vi "4 en linea.vi"() -> ()   [LabVIEW 2021]
panel:
  in  "OK Button":bool
  out "verde":bool
  in  "col7":bool
  in  "col6":bool
  in  "col5":bool
  in  "col4":bool
  in  "col3":bool
  in  "col2":bool
  in  "col1":bool
  in  "Ring 42":u16(ring)
  in  "Ring 41":u16(ring)
  in  "Ring 40":u16(ring)
  in  "Ring 39":u16(ring)
  in  "Ring 38":u16(ring)
  in  "Ring 37":u16(ring)
  in  "Ring 36":u16(ring)
  in  "Ring 35":u16(ring)
  in  "Ring 34":u16(ring)
  in  "Ring 33":u16(ring)
  in  "Ring 32":u16(ring)
  in  "Ring 31":u16(ring)
  in  "Ring 30":u16(ring)
  in  "Ring 29":u16(ring)
  in  "Ring 28":u16(ring)
  in  "Ring 27":u16(ring)
  in  "Ring 26":u16(ring)
  in  "Ring 25":u16(ring)
  in  "Ring 24":u16(ring)
  in  "Ring 23":u16(ring)
  in  "Ring 22":u16(ring)
  in  "Ring 21":u16(ring)
  in  "Ring 20":u16(ring)
  in  "Ring 19":u16(ring)
  in  "Ring 18":u16(ring)
  in  "Ring 17":u16(ring)
  in  "Ring 16":u16(ring)
  in  "Ring 15":u16(ring)
  in  "Ring 14":u16(ring)
  in  "Ring 13":u16(ring)
  in  "Ring 12":u16(ring)
  in  "Ring 11":u16(ring)
  in  "Ring 10":u16(ring)
  in  "Ring 9":u16(ring)
  in  "Ring 8":u16(ring)
  in  "Ring 7":u16(ring)
  in  "Ring 6":u16(ring)
  in  "Ring 5":u16(ring)
  in  "Ring 4":u16(ring)
  in  "Ring 3":u16(ring)
  in  "Ring 2":u16(ring)
  in  "Ring 1":u16(ring)
  # "4 EN LINEA"
  # "TURNO"
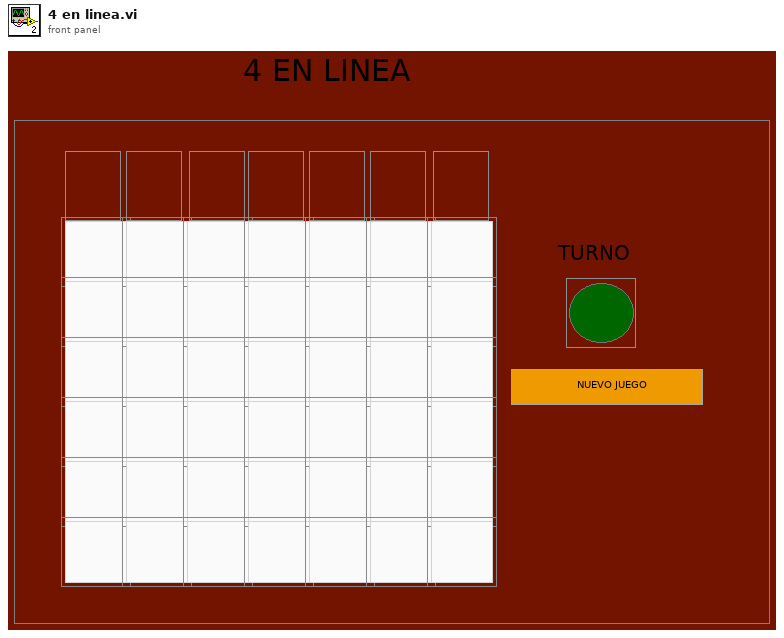
[diagram p1: front panel]
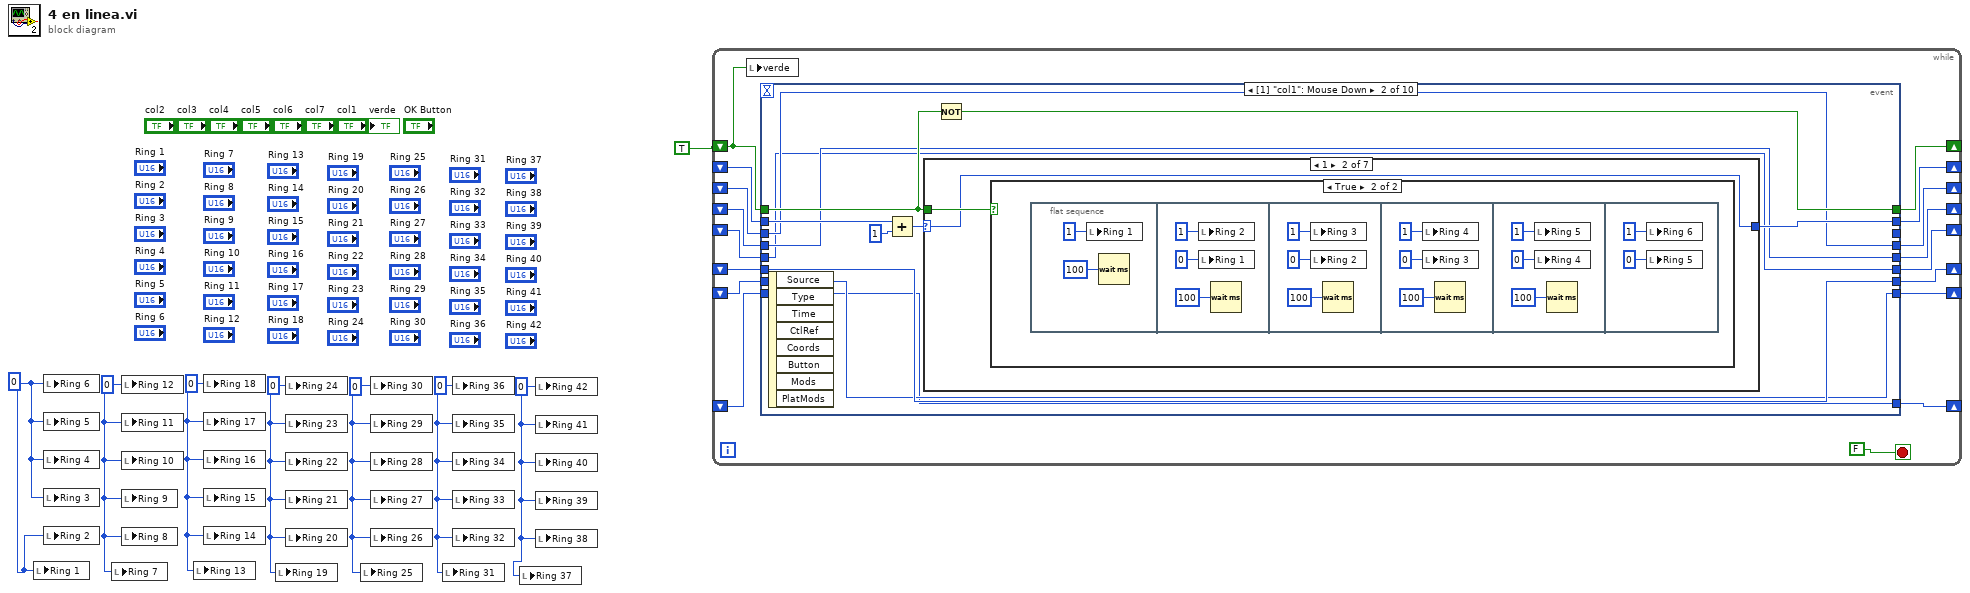
[diagram p0: block diagram]
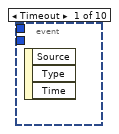
[diagram p2: hidden frame]
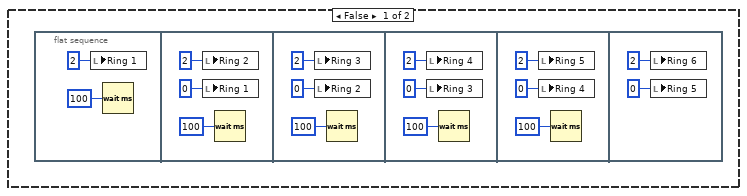
[diagram p4: hidden frame]
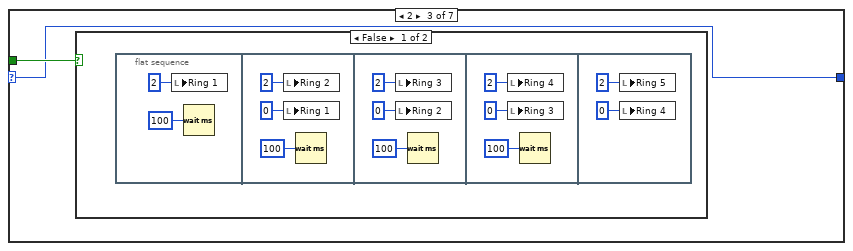
[diagram p5: hidden frame]
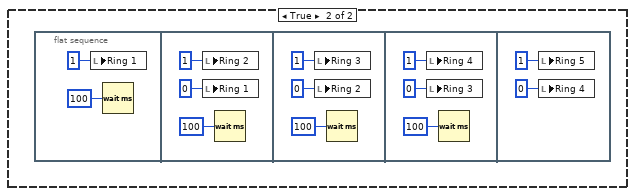
[diagram p6: hidden frame]
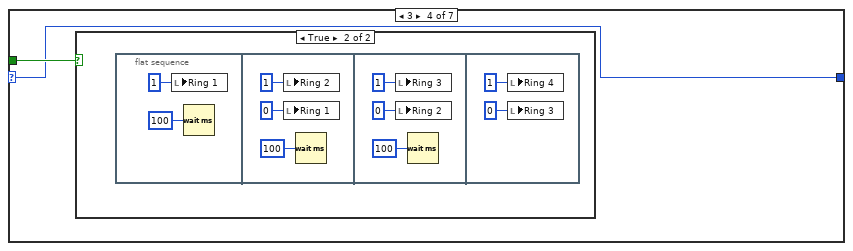
[diagram p7: hidden frame]
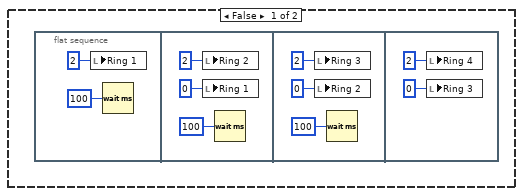
[diagram p8: hidden frame]
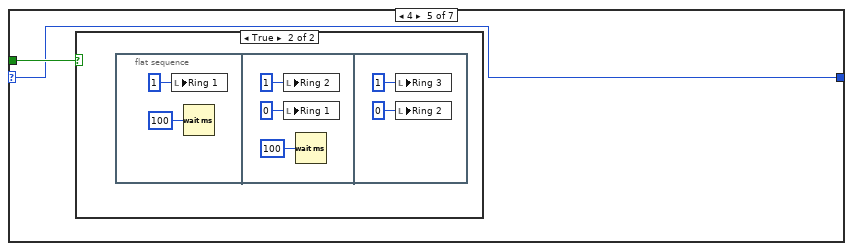
[diagram p9: hidden frame]
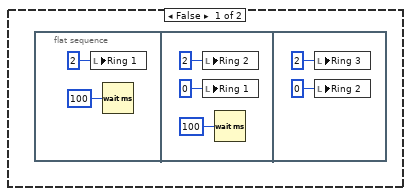
[diagram p10: hidden frame]
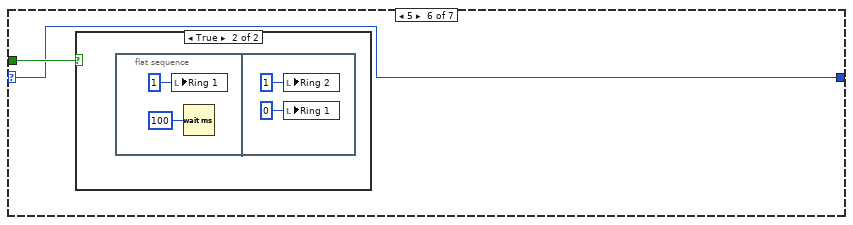
[diagram p11: hidden frame]
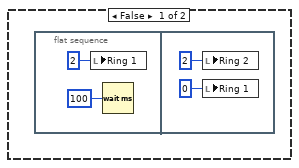
[diagram p12: hidden frame]
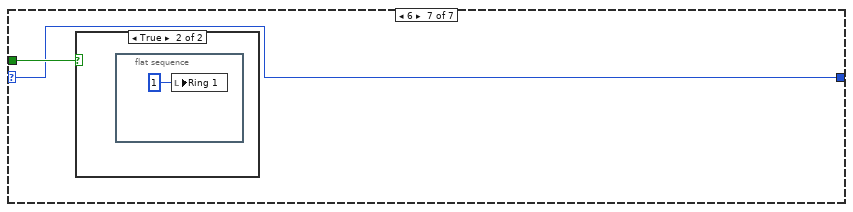
[diagram p13: hidden frame]
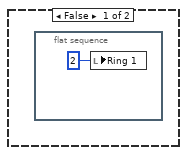
[diagram p14: hidden frame]
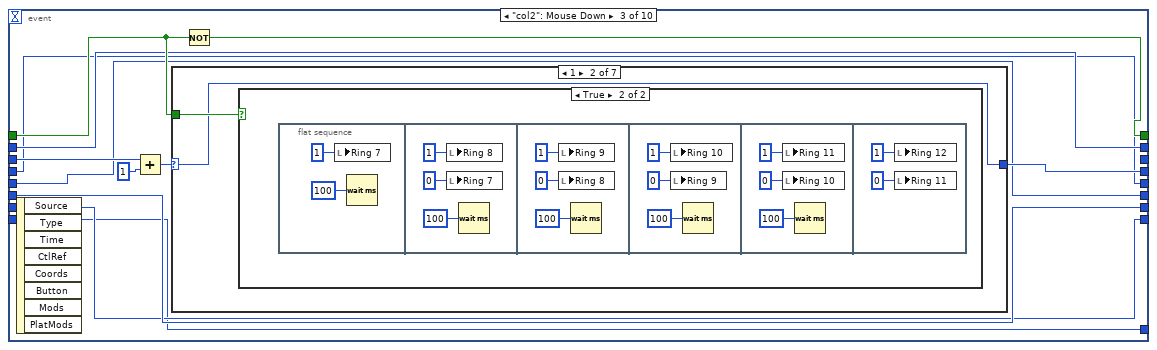
[diagram p15: hidden frame]
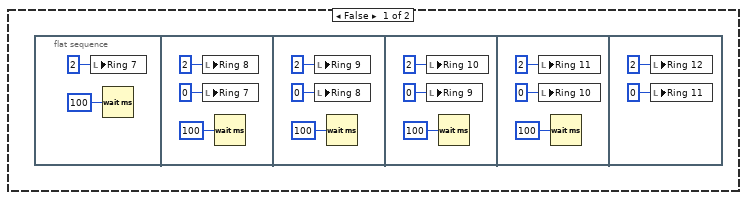
[diagram p17: hidden frame]
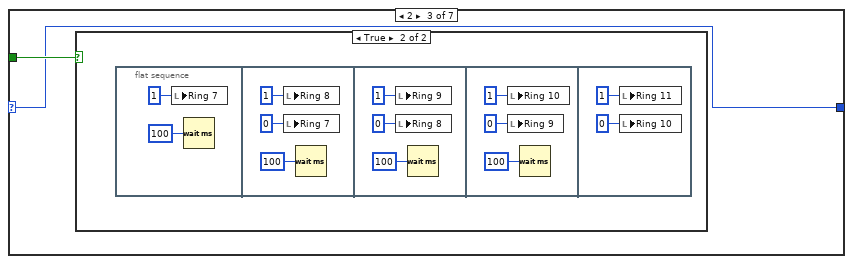
[diagram p18: hidden frame]
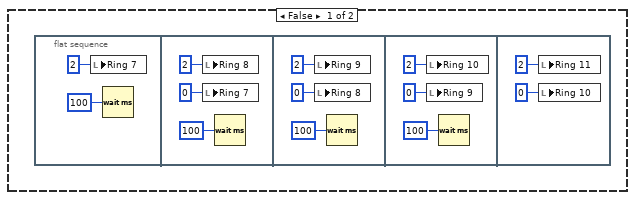
[diagram p19: hidden frame]
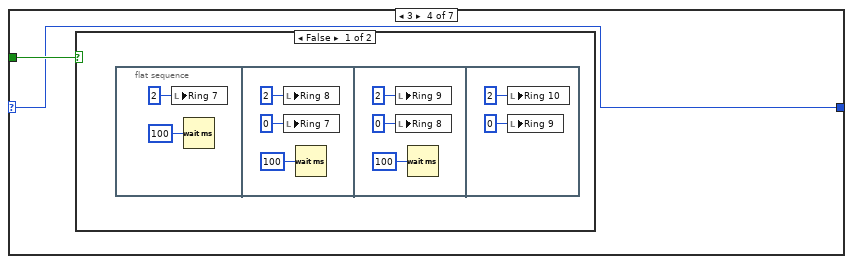
[diagram p20: hidden frame]
diagram:
  w2 = u16 0 ("Ring 42")
  w3 = u16 0 ("Ring 36")
  w4 = u16 0 ("Ring 30")
  w5 = u16 0 ("Ring 24")
  w6 = u16 0 ("Ring 18")
  w7 = u16 0 ("Ring 12")
  w8 = 0
  n1 = local write "Ring 1"(w8) -> ()
  n2 = local write "Ring 6"(w8) -> ()
  n3 = local write "Ring 5"(w8) -> ()
  n4 = local write "Ring 4"(w8) -> ()
  n5 = local write "Ring 3"(w8) -> ()
  n6 = local write "Ring 2"(w8) -> ()
  n7 = local write "Ring 7"(w7) -> ()
  n8 = local write "Ring 12"(w7) -> ()
  n9 = local write "Ring 11"(w7) -> ()
  n10 = local write "Ring 10"(w7) -> ()
  n11 = local write "Ring 9"(w7) -> ()
  n12 = local write "Ring 8"(w7) -> ()
  n13 = local write "Ring 13"(w6) -> ()
  n14 = local write "Ring 18"(w6) -> ()
  n15 = local write "Ring 17"(w6) -> ()
  n16 = local write "Ring 16"(w6) -> ()
  n17 = local write "Ring 15"(w6) -> ()
  n18 = local write "Ring 14"(w6) -> ()
  n19 = local write "Ring 19"(w5) -> ()
  n20 = local write "Ring 24"(w5) -> ()
  n21 = local write "Ring 23"(w5) -> ()
  n22 = local write "Ring 22"(w5) -> ()
  n23 = local write "Ring 21"(w5) -> ()
  n24 = local write "Ring 20"(w5) -> ()
  n25 = local write "Ring 25"(w4) -> ()
  n26 = local write "Ring 30"(w4) -> ()
  n27 = local write "Ring 29"(w4) -> ()
  n28 = local write "Ring 28"(w4) -> ()
  n29 = local write "Ring 27"(w4) -> ()
  n30 = local write "Ring 26"(w4) -> ()
  n31 = local write "Ring 31"(w3) -> ()
  n32 = local write "Ring 36"(w3) -> ()
  n33 = local write "Ring 35"(w3) -> ()
  n34 = local write "Ring 34"(w3) -> ()
  n35 = local write "Ring 33"(w3) -> ()
  n36 = local write "Ring 32"(w3) -> ()
  n37 = local write "Ring 37"(w2) -> ()
  n38 = local write "Ring 42"(w2) -> ()
  n39 = local write "Ring 41"(w2) -> ()
  n40 = local write "Ring 40"(w2) -> ()
  n41 = local write "Ring 39"(w2) -> ()
  n42 = local write "Ring 38"(w2) -> ()
  n43 = while {
    shift-right: [w24] -> _
    shift-left: TRUE -> [w9]
    shift-right: [w23] -> _
    shift-left: _ -> [w21]
    shift-right: [w22] -> _
    shift-left: _ -> [w20]
    shift-right: [w19] -> _
    shift-left: _ -> [w17]
    shift-right: [w18] -> _
    shift-left: _ -> [w16]
    shift-right: [w14] -> _
    shift-left: _ -> [w15]
    shift-right: [w12] -> _
    shift-left: _ -> [w13]
    shift-right: [w10] -> _
    shift-left: _ -> [w11]
    stop <- FALSE stop-if-true
    n44 = local write "verde"(w9) -> ()
    n45 = event shown="[1] \"col1\": Mouse Down" {
      selector: _ -> [_ _ _ _ _ _ _ _ _ _]
      dyn-events: _ -> [_ _ _ _ _ _ _ _ _ _]
      timeout: _ -> [_ _ _ _ _ _ _ _ _ _]
      tunnel: w9 -> [_ w36 w163 w285 w411 w540 w668 w788 w915 _]
      tunnel: [_ w37 w164 w286 w410 w541 w667 w789 w915 _] -> w24
      tunnel: [_ w35 w158 w289 w414 w536 w666 w795 _ _] -> w23
      tunnel: [_ w31 w162 w290 w413 w537 w665 w794 w921 _] -> w22
      tunnel: w21 -> [_ w34 w158 w289 w414 w536 w666 w795 w922 _]
      tunnel: w20 -> [_ w31 w161 w290 w413 w537 w665 w794 w921 _]
      tunnel: [_ w30 w157 w291 w412 w538 w664 w793 w920 _] -> w19
      tunnel: [_ w29 w156 w283 w416 w539 w663 w792 w919 _] -> w18
      tunnel: w17 -> [_ w30 w157 w284 w412 w538 w664 w793 w920 _]
      tunnel: w16 -> [_ w29 w156 w283 w415 w539 w663 w792 w919 _]
      tunnel: w15 -> [_ w28 w155 w282 w409 w544 w662 w791 w918 _]
      tunnel: [_ w28 w155 w282 w409 w542 w662 w791 w918 _] -> w14
      tunnel: w13 -> [_ w27 w154 w281 w408 w535 w671 w790 w917 _]
      tunnel: [_ w27 w154 w281 w408 w535 w669 w790 w917 _] -> w12
      tunnel: w11 -> [_ w26 w153 w280 w407 w534 w661 w798 w916 _]
      tunnel: [_ w26 w153 w280 w407 w534 w661 w796 w916 _] -> w10
      tunnel: [_ _ _ _ _ _ _ _ w922 _] -> _
      event Timeout {
        n46 = event-data() -> ()  [unwired: 1 in, 3 out]
      }
      event "col1": Mouse Down {
        n47 = event-data() -> ()  [unwired: 1 in, 8 out]
        n48 = Add(x=w34, y=1) -> (x+y=w33:i32)
        n49 = case shown="1" w33 {
          selector: w33 -> [w38 w39 w73 w101 w123 w139 w149]
          tunnel: w36 -> [_ w40 w74 w102 w124 w140 w150]
          tunnel: [w38 w39 w73 w101 w123 w139 w149] -> w35
          frame 0, Default {
          }
          frame 1 {
            n50 = case shown="True" w40 {
              frame False {
                n51 = flat-sequence {
                  frame #0 {
                    n52 = local write "Ring 1"(u16 2 ("Ring 1")) -> ()
                    n53 = Wait (ms)(milliseconds to wait=u32 100) -> ()  [unwired: 1 out]
                  }
                  frame #1 {
                    n54 = local write "Ring 2"(u16 2 ("Ring 2")) -> ()
                    n55 = local write "Ring 1"(u16 0 ("Ring 1")) -> ()
                    n56 = Wait (ms)(milliseconds to wait=u32 100) -> ()  [unwired: 1 out]
                  }
                  frame #2 {
                    n57 = local write "Ring 3"(u16 2 ("Ring 3")) -> ()
                    n58 = local write "Ring 2"(u16 0 ("Ring 2")) -> ()
                    n59 = Wait (ms)(milliseconds to wait=u32 100) -> ()  [unwired: 1 out]
                  }
                  frame #3 {
                    n60 = local write "Ring 4"(u16 2 ("Ring 4")) -> ()
                    n61 = local write "Ring 3"(u16 0 ("Ring 3")) -> ()
                    n62 = Wait (ms)(milliseconds to wait=u32 100) -> ()  [unwired: 1 out]
                  }
                  frame #4 {
                    n63 = local write "Ring 5"(u16 2 ("Ring 5")) -> ()
                    n64 = local write "Ring 4"(u16 0 ("Ring 4")) -> ()
                    n65 = Wait (ms)(milliseconds to wait=u32 100) -> ()  [unwired: 1 out]
                  }
                  frame #5 {
                    n66 = local write "Ring 6"(u16 2 ("Ring 6")) -> ()
                    n67 = local write "Ring 5"(u16 0 ("Ring 5")) -> ()
                  }
                }
              }
              frame True {
                n68 = flat-sequence {
                  frame #0 {
                    n69 = local write "Ring 1"(u16 1 ("Ring 1")) -> ()
                    n70 = Wait (ms)(milliseconds to wait=u32 100) -> ()  [unwired: 1 out]
                  }
                  frame #1 {
                    n71 = local write "Ring 2"(u16 1 ("Ring 2")) -> ()
                    n72 = local write "Ring 1"(u16 0 ("Ring 1")) -> ()
                    n73 = Wait (ms)(milliseconds to wait=u32 100) -> ()  [unwired: 1 out]
                  }
                  frame #2 {
                    n74 = local write "Ring 3"(u16 1 ("Ring 3")) -> ()
                    n75 = local write "Ring 2"(u16 0 ("Ring 2")) -> ()
                    n76 = Wait (ms)(milliseconds to wait=u32 100) -> ()  [unwired: 1 out]
                  }
                  frame #3 {
                    n77 = local write "Ring 4"(u16 1 ("Ring 4")) -> ()
                    n78 = local write "Ring 3"(u16 0 ("Ring 3")) -> ()
                    n79 = Wait (ms)(milliseconds to wait=u32 100) -> ()  [unwired: 1 out]
                  }
                  frame #4 {
                    n80 = local write "Ring 5"(u16 1 ("Ring 5")) -> ()
                    n81 = local write "Ring 4"(u16 0 ("Ring 4")) -> ()
                    n82 = Wait (ms)(milliseconds to wait=u32 100) -> ()  [unwired: 1 out]
                  }
                  frame #5 {
                    n83 = local write "Ring 6"(u16 1 ("Ring 6")) -> ()
                    n84 = local write "Ring 5"(u16 0 ("Ring 5")) -> ()
                  }
                }
              }
            }
          }
          frame 2 {
            n85 = case shown="False" w74 {
              frame False {
                n86 = flat-sequence {
                  frame #0 {
                    n87 = local write "Ring 1"(u16 2 ("Ring 1")) -> ()
                    n88 = Wait (ms)(milliseconds to wait=u32 100) -> ()  [unwired: 1 out]
                  }
                  frame #1 {
                    n89 = local write "Ring 2"(u16 2 ("Ring 2")) -> ()
                    n90 = local write "Ring 1"(u16 0 ("Ring 1")) -> ()
                    n91 = Wait (ms)(milliseconds to wait=u32 100) -> ()  [unwired: 1 out]
                  }
                  frame #2 {
                    n92 = local write "Ring 3"(u16 2 ("Ring 3")) -> ()
                    n93 = local write "Ring 2"(u16 0 ("Ring 2")) -> ()
                    n94 = Wait (ms)(milliseconds to wait=u32 100) -> ()  [unwired: 1 out]
                  }
                  frame #3 {
                    n95 = local write "Ring 4"(u16 2 ("Ring 4")) -> ()
                    n96 = local write "Ring 3"(u16 0 ("Ring 3")) -> ()
                    n97 = Wait (ms)(milliseconds to wait=u32 100) -> ()  [unwired: 1 out]
                  }
                  frame #4 {
                    n98 = local write "Ring 5"(u16 2 ("Ring 5")) -> ()
                    n99 = local write "Ring 4"(u16 0 ("Ring 4")) -> ()
                  }
                }
              }
              frame True {
                n100 = flat-sequence {
                  frame #0 {
                    n101 = local write "Ring 1"(u16 1 ("Ring 1")) -> ()
                    n102 = Wait (ms)(milliseconds to wait=u32 100) -> ()  [unwired: 1 out]
                  }
                  frame #1 {
                    n103 = local write "Ring 2"(u16 1 ("Ring 2")) -> ()
                    n104 = local write "Ring 1"(u16 0 ("Ring 1")) -> ()
                    n105 = Wait (ms)(milliseconds to wait=u32 100) -> ()  [unwired: 1 out]
                  }
                  frame #2 {
                    n106 = local write "Ring 3"(u16 1 ("Ring 3")) -> ()
                    n107 = local write "Ring 2"(u16 0 ("Ring 2")) -> ()
                    n108 = Wait (ms)(milliseconds to wait=u32 100) -> ()  [unwired: 1 out]
                  }
                  frame #3 {
                    n109 = local write "Ring 4"(u16 1 ("Ring 4")) -> ()
                    n110 = local write "Ring 3"(u16 0 ("Ring 3")) -> ()
                    n111 = Wait (ms)(milliseconds to wait=u32 100) -> ()  [unwired: 1 out]
                  }
                  frame #4 {
                    n112 = local write "Ring 5"(u16 1 ("Ring 5")) -> ()
                    n113 = local write "Ring 4"(u16 0 ("Ring 4")) -> ()
                  }
                }
              }
            }
          }
          frame 3 {
            n114 = case shown="True" w102 {
              frame False {
                n115 = flat-sequence {
                  frame #0 {
                    n116 = local write "Ring 1"(u16 2 ("Ring 1")) -> ()
                    n117 = Wait (ms)(milliseconds to wait=u32 100) -> ()  [unwired: 1 out]
                  }
                  frame #1 {
                    n118 = local write "Ring 2"(u16 2 ("Ring 2")) -> ()
                    n119 = local write "Ring 1"(u16 0 ("Ring 1")) -> ()
                    n120 = Wait (ms)(milliseconds to wait=u32 100) -> ()  [unwired: 1 out]
                  }
                  frame #2 {
                    n121 = local write "Ring 3"(u16 2 ("Ring 3")) -> ()
                    n122 = local write "Ring 2"(u16 0 ("Ring 2")) -> ()
                    n123 = Wait (ms)(milliseconds to wait=u32 100) -> ()  [unwired: 1 out]
                  }
                  frame #3 {
                    n124 = local write "Ring 4"(u16 2 ("Ring 4")) -> ()
                    n125 = local write "Ring 3"(u16 0 ("Ring 3")) -> ()
                  }
                }
              }
              frame True {
                n126 = flat-sequence {
                  frame #0 {
                    n127 = local write "Ring 1"(u16 1 ("Ring 1")) -> ()
                    n128 = Wait (ms)(milliseconds to wait=u32 100) -> ()  [unwired: 1 out]
                  }
                  frame #1 {
                    n129 = local write "Ring 2"(u16 1 ("Ring 2")) -> ()
                    n130 = local write "Ring 1"(u16 0 ("Ring 1")) -> ()
                    n131 = Wait (ms)(milliseconds to wait=u32 100) -> ()  [unwired: 1 out]
                  }
                  frame #2 {
                    n132 = local write "Ring 3"(u16 1 ("Ring 3")) -> ()
                    n133 = local write "Ring 2"(u16 0 ("Ring 2")) -> ()
                    n134 = Wait (ms)(milliseconds to wait=u32 100) -> ()  [unwired: 1 out]
                  }
                  frame #3 {
                    n135 = local write "Ring 4"(u16 1 ("Ring 4")) -> ()
                    n136 = local write "Ring 3"(u16 0 ("Ring 3")) -> ()
                  }
                }
              }
            }
          }
          frame 4 {
            n137 = case shown="True" w124 {
              frame False {
                n138 = flat-sequence {
                  frame #0 {
                    n139 = local write "Ring 1"(u16 2 ("Ring 1")) -> ()
                    n140 = Wait (ms)(milliseconds to wait=u32 100) -> ()  [unwired: 1 out]
                  }
                  frame #1 {
                    n141 = local write "Ring 2"(u16 2 ("Ring 2")) -> ()
                    n142 = local write "Ring 1"(u16 0 ("Ring 1")) -> ()
                    n143 = Wait (ms)(milliseconds to wait=u32 100) -> ()  [unwired: 1 out]
                  }
                  frame #2 {
                    n144 = local write "Ring 3"(u16 2 ("Ring 3")) -> ()
                    n145 = local write "Ring 2"(u16 0 ("Ring 2")) -> ()
                  }
                }
              }
              frame True {
                n146 = flat-sequence {
                  frame #0 {
                    n147 = local write "Ring 1"(u16 1 ("Ring 1")) -> ()
                    n148 = Wait (ms)(milliseconds to wait=u32 100) -> ()  [unwired: 1 out]
                  }
                  frame #1 {
                    n149 = local write "Ring 2"(u16 1 ("Ring 2")) -> ()
                    n150 = local write "Ring 1"(u16 0 ("Ring 1")) -> ()
                    n151 = Wait (ms)(milliseconds to wait=u32 100) -> ()  [unwired: 1 out]
                  }
                  frame #2 {
                    n152 = local write "Ring 3"(u16 1 ("Ring 3")) -> ()
                    n153 = local write "Ring 2"(u16 0 ("Ring 2")) -> ()
                  }
                }
              }
            }
          }
          frame 5 {
            n154 = case shown="True" w140 {
              frame False {
                n155 = flat-sequence {
                  frame #0 {
                    n156 = local write "Ring 1"(u16 2 ("Ring 1")) -> ()
                    n157 = Wait (ms)(milliseconds to wait=u32 100) -> ()  [unwired: 1 out]
                  }
                  frame #1 {
                    n158 = local write "Ring 2"(u16 2 ("Ring 2")) -> ()
                    n159 = local write "Ring 1"(u16 0 ("Ring 1")) -> ()
                  }
                }
              }
              frame True {
                n160 = flat-sequence {
                  frame #0 {
                    n161 = local write "Ring 1"(u16 1 ("Ring 1")) -> ()
                    n162 = Wait (ms)(milliseconds to wait=u32 100) -> ()  [unwired: 1 out]
                  }
                  frame #1 {
                    n163 = local write "Ring 2"(u16 1 ("Ring 2")) -> ()
                    n164 = local write "Ring 1"(u16 0 ("Ring 1")) -> ()
                  }
                }
              }
            }
          }
          frame 6 {
            n165 = case shown="True" w150 {
              frame False {
                n166 = flat-sequence {
                  frame #0 {
                    n167 = local write "Ring 1"(u16 2 ("Ring 1")) -> ()
                  }
                }
              }
              frame True {
                n168 = flat-sequence {
                  frame #0 {
                    n169 = local write "Ring 1"(u16 1 ("Ring 1")) -> ()
                  }
                }
              }
            }
          }
        }
        n170 = Not(x=w36) -> (.not. x?=w37:bool)
      }
      event "col2": Mouse Down {
        n171 = event-data() -> ()  [unwired: 1 in, 8 out]
        n172 = Add(x=w161, y=1) -> (x+y=w160:i32)
        n173 = case shown="1" w160 {
          selector: w160 -> [w165 w166 w200 w228 w250 w266 w276]
          tunnel: w163 -> [_ w167 w201 w229 w251 w267 w277]
          tunnel: [w165 w166 w200 w228 w250 w266 w276] -> w162
          frame 0, Default {
          }
          frame 1 {
            n174 = case shown="True" w167 {
              frame False {
                n175 = flat-sequence {
                  frame #0 {
                    n176 = local write "Ring 7"(u16 2 ("Ring 1")) -> ()
                    n177 = Wait (ms)(milliseconds to wait=u32 100) -> ()  [unwired: 1 out]
                  }
                  frame #1 {
                    n178 = local write "Ring 8"(u16 2 ("Ring 2")) -> ()
                    n179 = local write "Ring 7"(u16 0 ("Ring 1")) -> ()
                    n180 = Wait (ms)(milliseconds to wait=u32 100) -> ()  [unwired: 1 out]
                  }
                  frame #2 {
                    n181 = local write "Ring 9"(u16 2 ("Ring 3")) -> ()
                    n182 = local write "Ring 8"(u16 0 ("Ring 2")) -> ()
                    n183 = Wait (ms)(milliseconds to wait=u32 100) -> ()  [unwired: 1 out]
                  }
                  frame #3 {
                    n184 = local write "Ring 10"(u16 2 ("Ring 4")) -> ()
                    n185 = local write "Ring 9"(u16 0 ("Ring 3")) -> ()
                    n186 = Wait (ms)(milliseconds to wait=u32 100) -> ()  [unwired: 1 out]
                  }
                  frame #4 {
                    n187 = local write "Ring 11"(u16 2 ("Ring 5")) -> ()
                    n188 = local write "Ring 10"(u16 0 ("Ring 4")) -> ()
                    n189 = Wait (ms)(milliseconds to wait=u32 100) -> ()  [unwired: 1 out]
                  }
                  frame #5 {
                    n190 = local write "Ring 12"(u16 2 ("Ring 6")) -> ()
                    n191 = local write "Ring 11"(u16 0 ("Ring 5")) -> ()
                  }
                }
              }
              frame True {
                n192 = flat-sequence {
                  frame #0 {
                    n193 = local write "Ring 7"(u16 1 ("Ring 1")) -> ()
                    n194 = Wait (ms)(milliseconds to wait=u32 100) -> ()  [unwired: 1 out]
                  }
                  frame #1 {
                    n195 = local write "Ring 8"(u16 1 ("Ring 2")) -> ()
                    n196 = local write "Ring 7"(u16 0 ("Ring 1")) -> ()
                    n197 = Wait (ms)(milliseconds to wait=u32 100) -> ()  [unwired: 1 out]
                  }
                  frame #2 {
                    n198 = local write "Ring 9"(u16 1 ("Ring 3")) -> ()
                    n199 = local write "Ring 8"(u16 0 ("Ring 2")) -> ()
                    n200 = Wait (ms)(milliseconds to wait=u32 100) -> ()  [unwired: 1 out]
                  }
                  frame #3 {
                    n201 = local write "Ring 10"(u16 1 ("Ring 4")) -> ()
                    n202 = local write "Ring 9"(u16 0 ("Ring 3")) -> ()
                    n203 = Wait (ms)(milliseconds to wait=u32 100) -> ()  [unwired: 1 out]
                  }
                  frame #4 {
                    n204 = local write "Ring 11"(u16 1 ("Ring 5")) -> ()
                    n205 = local write "Ring 10"(u16 0 ("Ring 4")) -> ()
                    n206 = Wait (ms)(milliseconds to wait=u32 100) -> ()  [unwired: 1 out]
                  }
                  frame #5 {
                    n207 = local write "Ring 12"(u16 1 ("Ring 6")) -> ()
                    n208 = local write "Ring 11"(u16 0 ("Ring 5")) -> ()
                  }
                }
              }
            }
          }
          frame 2 {
            n209 = case shown="True" w201 {
              frame False {
                n210 = flat-sequence {
                  frame #0 {
                    n211 = local write "Ring 7"(u16 2 ("Ring 1")) -> ()
                    n212 = Wait (ms)(milliseconds to wait=u32 100) -> ()  [unwired: 1 out]
                  }
                  frame #1 {
                    n213 = local write "Ring 8"(u16 2 ("Ring 2")) -> ()
                    n214 = local write "Ring 7"(u16 0 ("Ring 1")) -> ()
                    n215 = Wait (ms)(milliseconds to wait=u32 100) -> ()  [unwired: 1 out]
                  }
                  frame #2 {
                    n216 = local write "Ring 9"(u16 2 ("Ring 3")) -> ()
                    n217 = local write "Ring 8"(u16 0 ("Ring 2")) -> ()
                    n218 = Wait (ms)(milliseconds to wait=u32 100) -> ()  [unwired: 1 out]
                  }
                  frame #3 {
                    n219 = local write "Ring 10"(u16 2 ("Ring 4")) -> ()
                    n220 = local write "Ring 9"(u16 0 ("Ring 3")) -> ()
                    n221 = Wait (ms)(milliseconds to wait=u32 100) -> ()  [unwired: 1 out]
                  }
                  frame #4 {
                    n222 = local write "Ring 11"(u16 2 ("Ring 5")) -> ()
                    n223 = local write "Ring 10"(u16 0 ("Ring 4")) -> ()
                  }
                }
              }
              frame True {
                n224 = flat-sequence {
                  frame #0 {
                    n225 = local write "Ring 7"(u16 1 ("Ring 1")) -> ()
                    n226 = Wait (ms)(milliseconds to wait=u32 100) -> ()  [unwired: 1 out]
                  }
                  frame #1 {
                    n227 = local write "Ring 8"(u16 1 ("Ring 2")) -> ()
                    n228 = local write "Ring 7"(u16 0 ("Ring 1")) -> ()
                    n229 = Wait (ms)(milliseconds to wait=u32 100) -> ()  [unwired: 1 out]
                  }
                  frame #2 {
                    n230 = local write "Ring 9"(u16 1 ("Ring 3")) -> ()
                    n231 = local write "Ring 8"(u16 0 ("Ring 2")) -> ()
                    n232 = Wait (ms)(milliseconds to wait=u32 100) -> ()  [unwired: 1 out]
                  }
                  frame #3 {
                    n233 = local write "Ring 10"(u16 1 ("Ring 4")) -> ()
                    n234 = local write "Ring 9"(u16 0 ("Ring 3")) -> ()
                    n235 = Wait (ms)(milliseconds to wait=u32 100) -> ()  [unwired: 1 out]
                  }
                  frame #4 {
                    n236 = local write "Ring 11"(u16 1 ("Ring 5")) -> ()
                    n237 = local write "Ring 10"(u16 0 ("Ring 4")) -> ()
                  }
                }
              }
            }
          }
          frame 3 {
            n238 = case shown="False" w229 {
              frame False {
                n239 = flat-sequence {
                  frame #0 {
                    n240 = local write "Ring 7"(u16 2 ("Ring 1")) -> ()
                    n241 = Wait (ms)(milliseconds to wait=u32 100) -> ()  [unwired: 1 out]
                  }
                  frame #1 {
                    n242 = local write "Ring 8"(u16 2 ("Ring 2")) -> ()
                    n243 = local write "Ring 7"(u16 0 ("Ring 1")) -> ()
                    n244 = Wait (ms)(milliseconds to wait=u32 100) -> ()  [unwired: 1 out]
                  }
                  frame #2 {
                    n245 = local write "Ring 9"(u16 2 ("Ring 3")) -> ()
                    n246 = local write "Ring 8"(u16 0 ("Ring 2")) -> ()
                    n247 = Wait (ms)(milliseconds to wait=u32 100) -> ()  [unwired: 1 out]
                  }
                  frame #3 {
                    n248 = local write "Ring 10"(u16 2 ("Ring 4")) -> ()
                    n249 = local write "Ring 9"(u16 0 ("Ring 3")) -> ()
                  }
                }
              }
              frame True {
                n250 = flat-sequence {
                  frame #0 {
                    n251 = local write "Ring 7"(u16 1 ("Ring 1")) -> ()
                    n252 = Wait (ms)(milliseconds to wait=u32 100) -> ()  [unwired: 1 out]
                  }
                  frame #1 {
                    n253 = local write "Ring 8"(u16 1 ("Ring 2")) -> ()
                    n254 = local write "Ring 7"(u16 0 ("Ring 1")) -> ()
                    n255 = Wait (ms)(milliseconds to wait=u32 100) -> ()  [unwired: 1 out]
                  }
                  frame #2 {
                    n256 = local write "Ring 9"(u16 1 ("Ring 3")) -> ()
                    n257 = local write "Ring 8"(u16 0 ("Ring 2")) -> ()
                    n258 = Wait (ms)(milliseconds to wait=u32 100) -> ()  [unwired: 1 out]
                  }
                  frame #3 {
                    n259 = local write "Ring 10"(u16 1 ("Ring 4")) -> ()
                    n260 = local write "Ring 9"(u16 0 ("Ring 3")) -> ()
                  }
                }
              }
            }
          }
          frame 4 {
            n261 = case shown="True" w251 {
              frame False {
                n262 = flat-sequence {
                  frame #0 {
                    n263 = local write "Ring 7"(u16 2 ("Ring 1")) -> ()
                    n264 = Wait (ms)(milliseconds to wait=u32 100) -> ()  [unwired: 1 out]
                  }
                  frame #1 {
                    n265 = local write "Ring 8"(u16 2 ("Ring 2")) -> ()
                    n266 = local write "Ring 7"(u16 0 ("Ring 1")) -> ()
                    n267 = Wait (ms)(milliseconds to wait=u32 100) -> ()  [unwired: 1 out]
                  }
                  frame #2 {
                    n268 = local write "Ring 9"(u16 2 ("Ring 3")) -> ()
                    n269 = local write "Ring 8"(u16 0 ("Ring 2")) -> ()
                  }
                }
              }
              frame True {
                n270 = flat-sequence {
                  frame #0 {
                    n271 = local write "Ring 7"(u16 1 ("Ring 1")) -> ()
                    n272 = Wait (ms)(milliseconds to wait=u32 100) -> ()  [unwired: 1 out]
                  }
                  frame #1 {
                    n273 = local write "Ring 8"(u16 1 ("Ring 2")) -> ()
                    n274 = local write "Ring 7"(u16 0 ("Ring 1")) -> ()
                    n275 = Wait (ms)(milliseconds to wait=u32 100) -> ()  [unwired: 1 out]
                  }
                  frame #2 {
                    n276 = local write "Ring 9"(u16 1 ("Ring 3")) -> ()
                    n277 = local write "Ring 8"(u16 0 ("Ring 2")) -> ()
                  }
                }
              }
            }
          }
          frame 5 {
            n278 = case shown="True" w267 {
              frame False {
                n279 = flat-sequence {
                  frame #0 {
                    n280 = local write "Ring 7"(u16 2 ("Ring 1")) -> ()
                    n281 = Wait (ms)(milliseconds to wait=u32 100) -> ()  [unwired: 1 out]
                  }
                  frame #1 {
                    n282 = local write "Ring 8"(u16 2 ("Ring 2")) -> ()
                    n283 = local write "Ring 7"(u16 0 ("Ring 1")) -> ()
                  }
                }
              }
              frame True {
                n284 = flat-sequence {
                  frame #0 {
                    n285 = local write "Ring 7"(u16 1 ("Ring 1")) -> ()
                    n286 = Wait (ms)(milliseconds to wait=u32 100) -> ()  [unwired: 1 out]
                  }
                  frame #1 {
                    n287 = local write "Ring 8"(u16 1 ("Ring 2")) -> ()
                    n288 = local write "Ring 7"(u16 0 ("Ring 1")) -> ()
                  }
                }
              }
            }
          }
          frame 6 {
            n289 = case shown="False" w277 {
              frame False {
                n290 = flat-sequence {
                  frame #0 {
                    n291 = local write "Ring 7"(u16 2 ("Ring 1")) -> ()
                  }
                }
              }
              frame True {
                n292 = flat-sequence {
                  frame #0 {
                    n293 = local write "Ring 7"(u16 1 ("Ring 1")) -> ()
                  }
                }
              }
            }
          }
        }
        n294 = Not(x=w163) -> (.not. x?=w164:bool)
      }
      event "col3": Mouse Down {
        n295 = event-data() -> ()  [unwired: 1 in, 8 out]
        n296 = Add(x=w284, y=1) -> (x+y=w288:i32)
        n297 = case shown="1" w288 {
          selector: w288 -> [w292 w293 w327 w355 w377 w393 w403]
          tunnel: w285 -> [_ w294 w328 w356 w378 w394 w404]
          tunnel: [w292 w293 w327 w355 w377 w393 w403] -> w291
          frame 0, Default {
          }
          frame 1 {
            n298 = case shown="False" w294 {
              frame False {
                n299 = flat-sequence {
                  frame #0 {
                    n300 = local write "Ring 13"(u16 2 ("Ring 1")) -> ()
                    n301 = Wait (ms)(milliseconds to wait=u32 100) -> ()  [unwired: 1 out]
                  }
                  frame #1 {
                    n302 = local write "Ring 14"(u16 2 ("Ring 2")) -> ()
                    n303 = local write "Ring 13"(u16 0 ("Ring 1")) -> ()
                    n304 = Wait (ms)(milliseconds to wait=u32 100) -> ()  [unwired: 1 out]
                  }
                  frame #2 {
                    n305 = local write "Ring 15"(u16 2 ("Ring 3")) -> ()
                    n306 = local write "Ring 14"(u16 0 ("Ring 2")) -> ()
                    n307 = Wait (ms)(milliseconds to wait=u32 100) -> ()  [unwired: 1 out]
                  }
                  frame #3 {
                    n308 = local write "Ring 16"(u16 2 ("Ring 4")) -> ()
                    n309 = local write "Ring 15"(u16 0 ("Ring 3")) -> ()
                    n310 = Wait (ms)(milliseconds to wait=u32 100) -> ()  [unwired: 1 out]
                  }
                  frame #4 {
                    n311 = local write "Ring 17"(u16 2 ("Ring 5")) -> ()
                    n312 = local write "Ring 16"(u16 0 ("Ring 4")) -> ()
                    n313 = Wait (ms)(milliseconds to wait=u32 100) -> ()  [unwired: 1 out]
                  }
                  frame #5 {
                    n314 = local write "Ring 18"(u16 2 ("Ring 6")) -> ()
                    n315 = local write "Ring 17"(u16 0 ("Ring 5")) -> ()
                  }
                }
              }
              frame True {
                n316 = flat-sequence {
                  frame #0 {
                    n317 = local write "Ring 13"(u16 1 ("Ring 1")) -> ()
                    n318 = Wait (ms)(milliseconds to wait=u32 100) -> ()  [unwired: 1 out]
                  }
                  frame #1 {
                    n319 = local write "Ring 14"(u16 1 ("Ring 2")) -> ()
                    n320 = local write "Ring 13"(u16 0 ("Ring 1")) -> ()
                    n321 = Wait (ms)(milliseconds to wait=u32 100) -> ()  [unwired: 1 out]
                  }
                  frame #2 {
                    n322 = local write "Ring 15"(u16 1 ("Ring 3")) -> ()
                    n323 = local write "Ring 14"(u16 0 ("Ring 2")) -> ()
                    n324 = Wait (ms)(milliseconds to wait=u32 100) -> ()  [unwired: 1 out]
                  }
                  frame #3 {
                    n325 = local write "Ring 16"(u16 1 ("Ring 4")) -> ()
                    n326 = local write "Ring 15"(u16 0 ("Ring 3")) -> ()
                    n327 = Wait (ms)(milliseconds to wait=u32 100) -> ()  [unwired: 1 out]
                  }
                  frame #4 {
                    n328 = local write "Ring 17"(u16 1 ("Ring 5")) -> ()
                    n329 = local write "Ring 16"(u16 0 ("Ring 4")) -> ()
                    n330 = Wait (ms)(milliseconds to wait=u32 100) -> ()  [unwired: 1 out]
                  }
                  frame #5 {
                    n331 = local write "Ring 18"(u16 1 ("Ring 6")) -> ()
                    n332 = local write "Ring 17"(u16 0 ("Ring 5")) -> ()
                  }
                }
              }
            }
          }
          frame 2 {
            n333 = case shown="True" w328 {
              frame False {
                n334 = flat-sequence {
                  frame #0 {
                    n335 = local write "Ring 13"(u16 2 ("Ring 1")) -> ()
                    n336 = Wait (ms)(milliseconds to wait=u32 100) -> ()  [unwired: 1 out]
                  }
                  frame #1 {
                    n337 = local write "Ring 14"(u16 2 ("Ring 2")) -> ()
                    n338 = local write "Ring 13"(u16 0 ("Ring 1")) -> ()
                    n339 = Wait (ms)(milliseconds to wait=u32 100) -> ()  [unwired: 1 out]
                  }
                  frame #2 {
                    n340 = local write "Ring 15"(u16 2 ("Ring 3")) -> ()
                    n341 = local write "Ring 14"(u16 0 ("Ring 2")) -> ()
                    n342 = Wait (ms)(milliseconds to wait=u32 100) -> ()  [unwired: 1 out]
                  }
                  frame #3 {
                    n343 = local write "Ring 16"(u16 2 ("Ring 4")) -> ()
                    n344 = local write "Ring 15"(u16 0 ("Ring 3")) -> ()
                    n345 = Wait (ms)(milliseconds to wait=u32 100) -> ()  [unwired: 1 out]
                  }
                  frame #4 {
                    n346 = local write "Ring 17"(u16 2 ("Ring 5")) -> ()
                    n347 = local write "Ring 16"(u16 0 ("Ring 4")) -> ()
                  }
                }
              }
              frame True {
                n348 = flat-sequence {
                  frame #0 {
                    n349 = local write "Ring 13"(u16 1 ("Ring 1")) -> ()
                    n350 = Wait (ms)(milliseconds to wait=u32 100) -> ()  [unwired: 1 out]
                  }
                  frame #1 {
                    n351 = local write "Ring 14"(u16 1 ("Ring 2")) -> ()
                    n352 = local write "Ring 13"(u16 0 ("Ring 1")) -> ()
                    n353 = Wait (ms)(milliseconds to wait=u32 100) -> ()  [unwired: 1 out]
                  }
                  frame #2 {
                    n354 = local write "Ring 15"(u16 1 ("Ring 3")) -> ()
                    n355 = local write "Ring 14"(u16 0 ("Ring 2")) -> ()
                    n356 = Wait (ms)(milliseconds to wait=u32 100) -> ()  [unwired: 1 out]
                  }
                  frame #3 {
                    n357 = local write "Ring 16"(u16 1 ("Ring 4")) -> ()
                    n358 = local write "Ring 15"(u16 0 ("Ring 3")) -> ()
                    n359 = Wait (ms)(milliseconds to wait=u32 100) -> ()  [unwired: 1 out]
                  }
                  frame #4 {
                    n360 = local write "Ring 17"(u16 1 ("Ring 5")) -> ()
                    n361 = local write "Ring 16"(u16 0 ("Ring 4")) -> ()
                  }
                }
              }
            }
          }
          frame 3 {
            n362 = case shown="True" w356 {
              frame False {
                n363 = flat-sequence {
                  frame #0 {
                    n364 = local write "Ring 13"(u16 2 ("Ring 1")) -> ()
                    n365 = Wait (ms)(milliseconds to wait=u32 100) -> ()  [unwired: 1 out]
                  }
                  frame #1 {
                    n366 = local write "Ring 14"(u16 2 ("Ring 2")) -> ()
                    n367 = local write "Ring 13"(u16 0 ("Ring 1")) -> ()
                    n368 = Wait (ms)(milliseconds to wait=u32 100) -> ()  [unwired: 1 out]
                  }
                  frame #2 {
                    n369 = local write "Ring 15"(u16 2 ("Ring 3")) -> ()
                    n370 = local write "Ring 14"(u16 0 ("Ring 2")) -> ()
                    n371 = Wait (ms)(milliseconds to wait=u32 100) -> ()  [unwired: 1 out]
                  }
                  frame #3 {
                    n372 = local write "Ring 16"(u16 2 ("Ring 4")) -> ()
                    n373 = local write "Ring 15"(u16 0 ("Ring 3")) -> ()
                  }
                }
              }
              frame True {
                n374 = flat-sequence {
                  frame #0 {
                    n375 = local write "Ring 13"(u16 1 ("Ring 1")) -> ()
                    n376 = Wait (ms)(milliseconds to wait=u32 100) -> ()  [unwired: 1 out]
                  }
                  frame #1 {
                    n377 = local write "Ring 14"(u16 1 ("Ring 2")) -> ()
                    n378 = local write "Ring 13"(u16 0 ("Ring 1")) -> ()
                    n379 = Wait (ms)(milliseconds to wait=u32 100) -> ()  [unwired: 1 out]
                  }
                  frame #2 {
                    n380 = local write "Ring 15"(u16 1 ("Ring 3")) -> ()
                    n381 = local write "Ring 14"(u16 0 ("Ring 2")) -> ()
                    n382 = Wait (ms)(milliseconds to wait=u32 100) -> ()  [unwired: 1 out]
                  }
                  frame #3 {
                    n383 = local write "Ring 16"(u16 1 ("Ring 4")) -> ()
                    n384 = local write "Ring 15"(u16 0 ("Ring 3")) -> ()
                  }
                }
              }
            }
          }
          frame 4 {
            n385 = case shown="False" w378 {
              frame False {
                n386 = flat-sequence {
                  frame #0 {
                    n387 = local write "Ring 13"(u16 2 ("Ring 1")) -> ()
                    n388 = Wait (ms)(milliseconds to wait=u32 100) -> ()  [unwired: 1 out]
                  }
                  frame #1 {
                    n389 = local write "Ring 14"(u16 2 ("Ring 2")) -> ()
                    n390 = local write "Ring 13"(u16 0 ("Ring 1")) -> ()
                    n391 = Wait (ms)(milliseconds to wait=u32 100) -> ()  [unwired: 1 out]
                  }
                  frame #2 {
                    n392 = local write "Ring 15"(u16 2 ("Ring 3")) -> ()
                    n393 = local write "Ring 14"(u16 0 ("Ring 2")) -> ()
                  }
                }
              }
              frame True {
                n394 = flat-sequence {
                  frame #0 {
                    n395 = local write "Ring 13"(u16 1 ("Ring 1")) -> ()
                    n396 = Wait (ms)(milliseconds to wait=u32 100) -> ()  [unwired: 1 out]
                  }
                  frame #1 {
                    n397 = local write "Ring 14"(u16 1 ("Ring 2")) -> ()
                    n398 = local write "Ring 13"(u16 0 ("Ring 1")) -> ()
                    n399 = Wait (ms)(milliseconds to wait=u32 100) -> ()  [unwired: 1 out]
                  }
                  frame #2 {
                    n400 = local write "Ring 15"(u16 1 ("Ring 3")) -> ()
                    n401 = local write "Ring 14"(u16 0 ("Ring 2")) -> ()
                  }
                }
              }
            }
          }
          frame 5 {
            n402 = case shown="False" w394 {
              frame False {
                n403 = flat-sequence {
                  frame #0 {
                    n404 = local write "Ring 13"(u16 2 ("Ring 1")) -> ()
                    n405 = Wait (ms)(milliseconds to wait=u32 100) -> ()  [unwired: 1 out]
                  }
                  frame #1 {
                    n406 = local write "Ring 14"(u16 2 ("Ring 2")) -> ()
                    n407 = local write "Ring 13"(u16 0 ("Ring 1")) -> ()
                  }
                }
              }
              frame True {
                n408 = flat-sequence {
                  frame #0 {
                    n409 = local write "Ring 13"(u16 1 ("Ring 1")) -> ()
                    n410 = Wait (ms)(milliseconds to wait=u32 100) -> ()  [unwired: 1 out]
                  }
                  frame #1 {
                    n411 = local write "Ring 14"(u16 1 ("Ring 2")) -> ()
                    n412 = local write "Ring 13"(u16 0 ("Ring 1")) -> ()
                  }
                }
              }
            }
          }
          frame 6 {
            n413 = case shown="True" w404 {
              frame False {
                n414 = flat-sequence {
                  frame #0 {
                    n415 = local write "Ring 13"(u16 2 ("Ring 1")) -> ()
                  }
                }
              }
              frame True {
                n416 = flat-sequence {
                  frame #0 {
                    n417 = local write "Ring 13"(u16 1 ("Ring 1")) -> ()
                  }
                }
              }
            }
          }
        }
        n418 = Not(x=w285) -> (.not. x?=w286:bool)
      }
      event "col4": Mouse Down {
        n419 = event-data() -> ()  [unwired: 1 in, 8 out]
        n420 = Add(x=w415, y=1) -> (x+y=w417:i32)
        n421 = case shown="6" w417 {
          selector: w417 -> [w419 w421 w455 w483 w505 w521 w531]
          tunnel: [w419 w421 w455 w483 w505 w521 w531] -> w416
          tunnel: w411 -> [_ w420 w454 w482 w504 w520 w530]
          frame 0, Default {
          }
          frame 1 {
            n422 = case shown="False" w420 {
              frame False {
                n423 = flat-sequence {
                  frame #0 {
                    n424 = local write "Ring 19"(u16 2 ("Ring 1")) -> ()
                    n425 = Wait (ms)(milliseconds to wait=u32 100) -> ()  [unwired: 1 out]
                  }
                  frame #1 {
                    n426 = local write "Ring 20"(u16 2 ("Ring 2")) -> ()
                    n427 = local write "Ring 19"(u16 0 ("Ring 1")) -> ()
                    n428 = Wait (ms)(milliseconds to wait=u32 100) -> ()  [unwired: 1 out]
                  }
                  frame #2 {
                    n429 = local write "Ring 21"(u16 2 ("Ring 3")) -> ()
                    n430 = local write "Ring 20"(u16 0 ("Ring 2")) -> ()
                    n431 = Wait (ms)(milliseconds to wait=u32 100) -> ()  [unwired: 1 out]
                  }
                  frame #3 {
                    n432 = local write "Ring 22"(u16 2 ("Ring 4")) -> ()
                    n433 = local write "Ring 21"(u16 0 ("Ring 3")) -> ()
                    n434 = Wait (ms)(milliseconds to wait=u32 100) -> ()  [unwired: 1 out]
                  }
                  frame #4 {
                    n435 = local write "Ring 23"(u16 2 ("Ring 5")) -> ()
                    n436 = local write "Ring 22"(u16 0 ("Ring 4")) -> ()
                    n437 = Wait (ms)(milliseconds to wait=u32 100) -> ()  [unwired: 1 out]
                  }
                  frame #5 {
                    n438 = local write "Ring 24"(u16 2 ("Ring 6")) -> ()
                    n439 = local write "Ring 23"(u16 0 ("Ring 5")) -> ()
                  }
                }
              }
              frame True {
                n440 = flat-sequence {
                  frame #0 {
                    n441 = local write "Ring 19"(u16 1 ("Ring 1")) -> ()
                    n442 = Wait (ms)(milliseconds to wait=u32 100) -> ()  [unwired: 1 out]
                  }
                  frame #1 {
                    n443 = local write "Ring 20"(u16 1 ("Ring 2")) -> ()
                    n444 = local write "Ring 19"(u16 0 ("Ring 1")) -> ()
                    n445 = Wait (ms)(milliseconds to wait=u32 100) -> ()  [unwired: 1 out]
                  }
                  frame #2 {
                    n446 = local write "Ring 21"(u16 1 ("Ring 3")) -> ()
                    n447 = local write "Ring 20"(u16 0 ("Ring 2")) -> ()
                    n448 = Wait (ms)(milliseconds to wait=u32 100) -> ()  [unwired: 1 out]
                  }
                  frame #3 {
                    n449 = local write "Ring 22"(u16 1 ("Ring 4")) -> ()
                    n450 = local write "Ring 21"(u16 0 ("Ring 3")) -> ()
                    n451 = Wait (ms)(milliseconds to wait=u32 100) -> ()  [unwired: 1 out]
                  }
                  frame #4 {
                    n452 = local write "Ring 23"(u16 1 ("Ring 5")) -> ()
                    n453 = local write "Ring 22"(u16 0 ("Ring 4")) -> ()
                    n454 = Wait (ms)(milliseconds to wait=u32 100) -> ()  [unwired: 1 out]
                  }
                  frame #5 {
                    n455 = local write "Ring 24"(u16 1 ("Ring 6")) -> ()
                    n456 = local write "Ring 23"(u16 0 ("Ring 5")) -> ()
                  }
                }
              }
            }
          }
          frame 2 {
            n457 = case shown="True" w454 {
              frame False {
                n458 = flat-sequence {
                  frame #0 {
                    n459 = local write "Ring 19"(u16 2 ("Ring 1")) -> ()
                    n460 = Wait (ms)(milliseconds to wait=u32 100) -> ()  [unwired: 1 out]
                  }
                  frame #1 {
                    n461 = local write "Ring 20"(u16 2 ("Ring 2")) -> ()
                    n462 = local write "Ring 19"(u16 0 ("Ring 1")) -> ()
                    n463 = Wait (ms)(milliseconds to wait=u32 100) -> ()  [unwired: 1 out]
                  }
                  frame #2 {
                    n464 = local write "Ring 21"(u16 2 ("Ring 3")) -> ()
                    n465 = local write "Ring 20"(u16 0 ("Ring 2")) -> ()
                    n466 = Wait (ms)(milliseconds to wait=u32 100) -> ()  [unwired: 1 out]
                  }
                  frame #3 {
                    n467 = local write "Ring 22"(u16 2 ("Ring 4")) -> ()
                    n468 = local write "Ring 21"(u16 0 ("Ring 3")) -> ()
                    n469 = Wait (ms)(milliseconds to wait=u32 100) -> ()  [unwired: 1 out]
                  }
                  frame #4 {
                    n470 = local write "Ring 23"(u16 2 ("Ring 5")) -> ()
                    n471 = local write "Ring 22"(u16 0 ("Ring 4")) -> ()
                  }
                }
              }
              frame True {
                n472 = flat-sequence {
                  frame #0 {
                    n473 = local write "Ring 19"(u16 1 ("Ring 1")) -> ()
                    n474 = Wait (ms)(milliseconds to wait=u32 100) -> ()  [unwired: 1 out]
                  }
                  frame #1 {
                    n475 = local write "Ring 20"(u16 1 ("Ring 2")) -> ()
                    n476 = local write "Ring 19"(u16 0 ("Ring 1")) -> ()
                    n477 = Wait (ms)(milliseconds to wait=u32 100) -> ()  [unwired: 1 out]
                  }
                  frame #2 {
                    n478 = local write "Ring 21"(u16 1 ("Ring 3")) -> ()
                    n479 = local write "Ring 20"(u16 0 ("Ring 2")) -> ()
                    n480 = Wait (ms)(milliseconds to wait=u32 100) -> ()  [unwired: 1 out]
                  }
                  frame #3 {
                    n481 = local write "Ring 22"(u16 1 ("Ring 4")) -> ()
                    n482 = local write "Ring 21"(u16 0 ("Ring 3")) -> ()
                    n483 = Wait (ms)(milliseconds to wait=u32 100) -> ()  [unwired: 1 out]
                  }
                  frame #4 {
                    n484 = local write "Ring 23"(u16 1 ("Ring 5")) -> ()
                    n485 = local write "Ring 22"(u16 0 ("Ring 4")) -> ()
                  }
                }
              }
            }
          }
          frame 3 {
            n486 = case shown="False" w482 {
              frame False {
                n487 = flat-sequence {
                  frame #0 {
                    n488 = local write "Ring 19"(u16 2 ("Ring 1")) -> ()
                    n489 = Wait (ms)(milliseconds to wait=u32 100) -> ()  [unwired: 1 out]
                  }
                  frame #1 {
                    n490 = local write "Ring 20"(u16 2 ("Ring 2")) -> ()
                    n491 = local write "Ring 19"(u16 0 ("Ring 1")) -> ()
                    n492 = Wait (ms)(milliseconds to wait=u32 100) -> ()  [unwired: 1 out]
                  }
                  frame #2 {
                    n493 = local write "Ring 21"(u16 2 ("Ring 3")) -> ()
                    n494 = local write "Ring 20"(u16 0 ("Ring 2")) -> ()
                    n495 = Wait (ms)(milliseconds to wait=u32 100) -> ()  [unwired: 1 out]
                  }
                  frame #3 {
                    n496 = local write "Ring 22"(u16 2 ("Ring 4")) -> ()
                    n497 = local write "Ring 21"(u16 0 ("Ring 3")) -> ()
                  }
                }
              }
              frame True {
                n498 = flat-sequence {
                  frame #0 {
                    n499 = local write "Ring 19"(u16 1 ("Ring 1")) -> ()
                    n500 = Wait (ms)(milliseconds to wait=u32 100) -> ()  [unwired: 1 out]
                  }
                  frame #1 {
                    n501 = local write "Ring 20"(u16 1 ("Ring 2")) -> ()
                    n502 = local write "Ring 19"(u16 0 ("Ring 1")) -> ()
                    n503 = Wait (ms)(milliseconds to wait=u32 100) -> ()  [unwired: 1 out]
                  }
                  frame #2 {
                    n504 = local write "Ring 21"(u16 1 ("Ring 3")) -> ()
                    n505 = local write "Ring 20"(u16 0 ("Ring 2")) -> ()
                    n506 = Wait (ms)(milliseconds to wait=u32 100) -> ()  [unwired: 1 out]
                  }
                  frame #3 {
                    n507 = local write "Ring 22"(u16 1 ("Ring 4")) -> ()
                    n508 = local write "Ring 21"(u16 0 ("Ring 3")) -> ()
                  }
                }
              }
            }
          }
          frame 4 {
            n509 = case shown="False" w504 {
              frame False {
                n510 = flat-sequence {
                  frame #0 {
                    n511 = local write "Ring 19"(u16 2 ("Ring 1")) -> ()
                    n512 = Wait (ms)(milliseconds to wait=u32 100) -> ()  [unwired: 1 out]
                  }
                  frame #1 {
                    n513 = local write "Ring 20"(u16 2 ("Ring 2")) -> ()
                    n514 = local write "Ring 19"(u16 0 ("Ring 1")) -> ()
                    n515 = Wait (ms)(milliseconds to wait=u32 100) -> ()  [unwired: 1 out]
                  }
                  frame #2 {
                    n516 = local write "Ring 21"(u16 2 ("Ring 3")) -> ()
                    n517 = local write "Ring 20"(u16 0 ("Ring 2")) -> ()
                  }
                }
              }
              frame True {
                n518 = flat-sequence {
                  frame #0 {
                    n519 = local write "Ring 19"(u16 1 ("Ring 1")) -> ()
                    n520 = Wait (ms)(milliseconds to wait=u32 100) -> ()  [unwired: 1 out]
                  }
                  frame #1 {
                    n521 = local write "Ring 20"(u16 1 ("Ring 2")) -> ()
                    n522 = local write "Ring 19"(u16 0 ("Ring 1")) -> ()
                    n523 = Wait (ms)(milliseconds to wait=u32 100) -> ()  [unwired: 1 out]
                  }
                  frame #2 {
                    n524 = local write "Ring 21"(u16 1 ("Ring 3")) -> ()
                    n525 = local write "Ring 20"(u16 0 ("Ring 2")) -> ()
                  }
                }
              }
            }
          }
          frame 5 {
            n526 = case shown="False" w520 {
              frame False {
                n527 = flat-sequence {
                  frame #0 {
                    n528 = local write "Ring 19"(u16 2 ("Ring 1")) -> ()
                    n529 = Wait (ms)(milliseconds to wait=u32 100) -> ()  [unwired: 1 out]
                  }
                  frame #1 {
                    n530 = local write "Ring 20"(u16 2 ("Ring 2")) -> ()
                    n531 = local write "Ring 19"(u16 0 ("Ring 1")) -> ()
                  }
                }
              }
              frame True {
                n532 = flat-sequence {
                  frame #0 {
                    n533 = local write "Ring 19"(u16 1 ("Ring 1")) -> ()
                    n534 = Wait (ms)(milliseconds to wait=u32 100) -> ()  [unwired: 1 out]
                  }
                  frame #1 {
                    n535 = local write "Ring 20"(u16 1 ("Ring 2")) -> ()
                    n536 = local write "Ring 19"(u16 0 ("Ring 1")) -> ()
                  }
                }
              }
            }
          }
          frame 6 {
            n537 = case shown="False" w530 {
              frame False {
                n538 = flat-sequence {
                  frame #0 {
                    n539 = local write "Ring 19"(u16 2 ("Ring 1")) -> ()
                  }
                }
              }
              frame True {
                n540 = flat-sequence {
                  frame #0 {
                    n541 = local write "Ring 19"(u16 1 ("Ring 1")) -> ()
                  }
                }
              }
            }
          }
        }
        n542 = Not(x=w411) -> (.not. x?=w410:bool)
      }
      event "col5": Mouse Down {
        n543 = event-data() -> ()  [unwired: 1 in, 8 out]
        n544 = Add(x=w544, y=1) -> (x+y=w543:i32)
        n545 = case shown="6" w543 {
          selector: w543 -> [w546 w548 w582 w610 w632 w648 w658]
          tunnel: [w546 w548 w582 w610 w632 w648 w658] -> w542
          tunnel: w540 -> [_ w547 w581 w609 w631 w647 w657]
          frame 0, Default {
          }
          frame 1 {
            n546 = case shown="False" w547 {
              frame False {
                n547 = flat-sequence {
                  frame #0 {
                    n548 = local write "Ring 25"(u16 2 ("Ring 1")) -> ()
                    n549 = Wait (ms)(milliseconds to wait=u32 100) -> ()  [unwired: 1 out]
                  }
                  frame #1 {
                    n550 = local write "Ring 26"(u16 2 ("Ring 2")) -> ()
                    n551 = local write "Ring 25"(u16 0 ("Ring 1")) -> ()
                    n552 = Wait (ms)(milliseconds to wait=u32 100) -> ()  [unwired: 1 out]
                  }
                  frame #2 {
                    n553 = local write "Ring 27"(u16 2 ("Ring 3")) -> ()
                    n554 = local write "Ring 26"(u16 0 ("Ring 2")) -> ()
                    n555 = Wait (ms)(milliseconds to wait=u32 100) -> ()  [unwired: 1 out]
                  }
                  frame #3 {
                    n556 = local write "Ring 28"(u16 2 ("Ring 4")) -> ()
                    n557 = local write "Ring 27"(u16 0 ("Ring 3")) -> ()
                    n558 = Wait (ms)(milliseconds to wait=u32 100) -> ()  [unwired: 1 out]
                  }
                  frame #4 {
                    n559 = local write "Ring 29"(u16 2 ("Ring 5")) -> ()
                    n560 = local write "Ring 28"(u16 0 ("Ring 4")) -> ()
                    n561 = Wait (ms)(milliseconds to wait=u32 100) -> ()  [unwired: 1 out]
                  }
                  frame #5 {
                    n562 = local write "Ring 30"(u16 2 ("Ring 6")) -> ()
                    n563 = local write "Ring 29"(u16 0 ("Ring 5")) -> ()
                  }
                }
              }
              frame True {
                n564 = flat-sequence {
                  frame #0 {
                    n565 = local write "Ring 25"(u16 1 ("Ring 1")) -> ()
                    n566 = Wait (ms)(milliseconds to wait=u32 100) -> ()  [unwired: 1 out]
                  }
                  frame #1 {
                    n567 = local write "Ring 26"(u16 1 ("Ring 2")) -> ()
                    n568 = local write "Ring 25"(u16 0 ("Ring 1")) -> ()
                    n569 = Wait (ms)(milliseconds to wait=u32 100) -> ()  [unwired: 1 out]
                  }
                  frame #2 {
                    n570 = local write "Ring 27"(u16 1 ("Ring 3")) -> ()
                    n571 = local write "Ring 26"(u16 0 ("Ring 2")) -> ()
                    n572 = Wait (ms)(milliseconds to wait=u32 100) -> ()  [unwired: 1 out]
                  }
                  frame #3 {
                    n573 = local write "Ring 28"(u16 1 ("Ring 4")) -> ()
                    n574 = local write "Ring 27"(u16 0 ("Ring 3")) -> ()
                    n575 = Wait (ms)(milliseconds to wait=u32 100) -> ()  [unwired: 1 out]
                  }
                  frame #4 {
                    n576 = local write "Ring 29"(u16 1 ("Ring 5")) -> ()
                    n577 = local write "Ring 28"(u16 0 ("Ring 4")) -> ()
                    n578 = Wait (ms)(milliseconds to wait=u32 100) -> ()  [unwired: 1 out]
                  }
                  frame #5 {
                    n579 = local write "Ring 30"(u16 1 ("Ring 6")) -> ()
                    n580 = local write "Ring 29"(u16 0 ("Ring 5")) -> ()
                  }
                }
              }
            }
          }
          frame 2 {
            n581 = case shown="False" w581 {
              frame False {
                n582 = flat-sequence {
                  frame #0 {
                    n583 = local write "Ring 25"(u16 2 ("Ring 1")) -> ()
                    n584 = Wait (ms)(milliseconds to wait=u32 100) -> ()  [unwired: 1 out]
                  }
                  frame #1 {
                    n585 = local write "Ring 26"(u16 2 ("Ring 2")) -> ()
                    n586 = local write "Ring 25"(u16 0 ("Ring 1")) -> ()
                    n587 = Wait (ms)(milliseconds to wait=u32 100) -> ()  [unwired: 1 out]
                  }
                  frame #2 {
                    n588 = local write "Ring 27"(u16 2 ("Ring 3")) -> ()
                    n589 = local write "Ring 26"(u16 0 ("Ring 2")) -> ()
                    n590 = Wait (ms)(milliseconds to wait=u32 100) -> ()  [unwired: 1 out]
                  }
                  frame #3 {
                    n591 = local write "Ring 28"(u16 2 ("Ring 4")) -> ()
                    n592 = local write "Ring 27"(u16 0 ("Ring 3")) -> ()
                    n593 = Wait (ms)(milliseconds to wait=u32 100) -> ()  [unwired: 1 out]
                  }
                  frame #4 {
                    n594 = local write "Ring 29"(u16 2 ("Ring 5")) -> ()
                    n595 = local write "Ring 28"(u16 0 ("Ring 4")) -> ()
                  }
                }
              }
              frame True {
                n596 = flat-sequence {
                  frame #0 {
                    n597 = local write "Ring 25"(u16 1 ("Ring 1")) -> ()
                    n598 = Wait (ms)(milliseconds to wait=u32 100) -> ()  [unwired: 1 out]
                  }
                  frame #1 {
                    n599 = local write "Ring 26"(u16 1 ("Ring 2")) -> ()
                    n600 = local write "Ring 25"(u16 0 ("Ring 1")) -> ()
                    n601 = Wait (ms)(milliseconds to wait=u32 100) -> ()  [unwired: 1 out]
                  }
                  frame #2 {
                    n602 = local write "Ring 27"(u16 1 ("Ring 3")) -> ()
                    n603 = local write "Ring 26"(u16 0 ("Ring 2")) -> ()
                    n604 = Wait (ms)(milliseconds to wait=u32 100) -> ()  [unwired: 1 out]
                  }
                  frame #3 {
                    n605 = local write "Ring 28"(u16 1 ("Ring 4")) -> ()
                    n606 = local write "Ring 27"(u16 0 ("Ring 3")) -> ()
                    n607 = Wait (ms)(milliseconds to wait=u32 100) -> ()  [unwired: 1 out]
                  }
                  frame #4 {
                    n608 = local write "Ring 29"(u16 1 ("Ring 5")) -> ()
                    n609 = local write "Ring 28"(u16 0 ("Ring 4")) -> ()
                  }
                }
              }
            }
          }
          frame 3 {
            n610 = case shown="False" w609 {
              frame False {
                n611 = flat-sequence {
                  frame #0 {
                    n612 = local write "Ring 25"(u16 2 ("Ring 1")) -> ()
                    n613 = Wait (ms)(milliseconds to wait=u32 100) -> ()  [unwired: 1 out]
                  }
                  frame #1 {
                    n614 = local write "Ring 26"(u16 2 ("Ring 2")) -> ()
                    n615 = local write "Ring 25"(u16 0 ("Ring 1")) -> ()
                    n616 = Wait (ms)(milliseconds to wait=u32 100) -> ()  [unwired: 1 out]
                  }
                  frame #2 {
                    n617 = local write "Ring 27"(u16 2 ("Ring 3")) -> ()
                    n618 = local write "Ring 26"(u16 0 ("Ring 2")) -> ()
                    n619 = Wait (ms)(milliseconds to wait=u32 100) -> ()  [unwired: 1 out]
                  }
                  frame #3 {
                    n620 = local write "Ring 28"(u16 2 ("Ring 4")) -> ()
                    n621 = local write "Ring 27"(u16 0 ("Ring 3")) -> ()
                  }
                }
              }
              frame True {
                n622 = flat-sequence {
                  frame #0 {
                    n623 = local write "Ring 25"(u16 1 ("Ring 1")) -> ()
                    n624 = Wait (ms)(milliseconds to wait=u32 100) -> ()  [unwired: 1 out]
                  }
                  frame #1 {
                    n625 = local write "Ring 26"(u16 1 ("Ring 2")) -> ()
                    n626 = local write "Ring 25"(u16 0 ("Ring 1")) -> ()
                    n627 = Wait (ms)(milliseconds to wait=u32 100) -> ()  [unwired: 1 out]
                  }
                  frame #2 {
                    n628 = local write "Ring 27"(u16 1 ("Ring 3")) -> ()
                    n629 = local write "Ring 26"(u16 0 ("Ring 2")) -> ()
                    n630 = Wait (ms)(milliseconds to wait=u32 100) -> ()  [unwired: 1 out]
                  }
                  frame #3 {
                    n631 = local write "Ring 28"(u16 1 ("Ring 4")) -> ()
                    n632 = local write "Ring 27"(u16 0 ("Ring 3")) -> ()
                  }
                }
              }
            }
          }
          frame 4 {
            n633 = case shown="False" w631 {
              frame False {
                n634 = flat-sequence {
                  frame #0 {
                    n635 = local write "Ring 25"(u16 2 ("Ring 1")) -> ()
                    n636 = Wait (ms)(milliseconds to wait=u32 100) -> ()  [unwired: 1 out]
                  }
                  frame #1 {
                    n637 = local write "Ring 26"(u16 2 ("Ring 2")) -> ()
                    n638 = local write "Ring 25"(u16 0 ("Ring 1")) -> ()
                    n639 = Wait (ms)(milliseconds to wait=u32 100) -> ()  [unwired: 1 out]
                  }
                  frame #2 {
                    n640 = local write "Ring 27"(u16 2 ("Ring 3")) -> ()
                    n641 = local write "Ring 26"(u16 0 ("Ring 2")) -> ()
                  }
                }
              }
              frame True {
                n642 = flat-sequence {
                  frame #0 {
                    n643 = local write "Ring 25"(u16 1 ("Ring 1")) -> ()
                    n644 = Wait (ms)(milliseconds to wait=u32 100) -> ()  [unwired: 1 out]
                  }
                  frame #1 {
                    n645 = local write "Ring 26"(u16 1 ("Ring 2")) -> ()
                    n646 = local write "Ring 25"(u16 0 ("Ring 1")) -> ()
                    n647 = Wait (ms)(milliseconds to wait=u32 100) -> ()  [unwired: 1 out]
                  }
                  frame #2 {
                    n648 = local write "Ring 27"(u16 1 ("Ring 3")) -> ()
                    n649 = local write "Ring 26"(u16 0 ("Ring 2")) -> ()
                  }
                }
              }
            }
          }
          frame 5 {
            n650 = case shown="True" w647 {
              frame False {
                n651 = flat-sequence {
                  frame #0 {
                    n652 = local write "Ring 25"(u16 2 ("Ring 1")) -> ()
                    n653 = Wait (ms)(milliseconds to wait=u32 100) -> ()  [unwired: 1 out]
                  }
                  frame #1 {
                    n654 = local write "Ring 26"(u16 2 ("Ring 2")) -> ()
                    n655 = local write "Ring 25"(u16 0 ("Ring 1")) -> ()
                  }
                }
              }
              frame True {
                n656 = flat-sequence {
                  frame #0 {
                    n657 = local write "Ring 25"(u16 1 ("Ring 1")) -> ()
                    n658 = Wait (ms)(milliseconds to wait=u32 100) -> ()  [unwired: 1 out]
                  }
                  frame #1 {
                    n659 = local write "Ring 26"(u16 1 ("Ring 2")) -> ()
                    n660 = local write "Ring 25"(u16 0 ("Ring 1")) -> ()
                  }
                }
              }
            }
          }
          frame 6 {
            n661 = case shown="True" w657 {
              frame False {
                n662 = flat-sequence {
                  frame #0 {
                    n663 = local write "Ring 25"(u16 2 ("Ring 1")) -> ()
                  }
                }
              }
              frame True {
                n664 = flat-sequence {
                  frame #0 {
                    n665 = local write "Ring 25"(u16 1 ("Ring 1")) -> ()
                  }
                }
              }
            }
          }
        }
        n666 = Not(x=w540) -> (.not. x?=w541:bool)
      }
      event "col6": Mouse Down {
        n667 = event-data() -> ()  [unwired: 1 in, 8 out]
        n668 = Add(x=w671, y=1) -> (x+y=w670:i32)
        n669 = case shown="1" w670 {
          selector: w670 -> [w673 w675 w709 w737 w759 w775 w785]
          tunnel: [w673 w675 w709 w737 w759 w775 w785] -> w669
          tunnel: w668 -> [_ w674 w708 w736 w758 w774 w784]
          frame 0, Default {
          }
          frame 1 {
            n670 = case shown="True" w674 {
              frame False {
                n671 = flat-sequence {
                  frame #0 {
                    n672 = local write "Ring 31"(u16 2 ("Ring 1")) -> ()
                    n673 = Wait (ms)(milliseconds to wait=u32 100) -> ()  [unwired: 1 out]
                  }
                  frame #1 {
                    n674 = local write "Ring 32"(u16 2 ("Ring 2")) -> ()
                    n675 = local write "Ring 31"(u16 0 ("Ring 1")) -> ()
                    n676 = Wait (ms)(milliseconds to wait=u32 100) -> ()  [unwired: 1 out]
                  }
                  frame #2 {
                    n677 = local write "Ring 33"(u16 2 ("Ring 3")) -> ()
                    n678 = local write "Ring 32"(u16 0 ("Ring 2")) -> ()
                    n679 = Wait (ms)(milliseconds to wait=u32 100) -> ()  [unwired: 1 out]
                  }
                  frame #3 {
                    n680 = local write "Ring 34"(u16 2 ("Ring 4")) -> ()
                    n681 = local write "Ring 33"(u16 0 ("Ring 3")) -> ()
                    n682 = Wait (ms)(milliseconds to wait=u32 100) -> ()  [unwired: 1 out]
                  }
                  frame #4 {
                    n683 = local write "Ring 35"(u16 2 ("Ring 5")) -> ()
                    n684 = local write "Ring 34"(u16 0 ("Ring 4")) -> ()
                    n685 = Wait (ms)(milliseconds to wait=u32 100) -> ()  [unwired: 1 out]
                  }
                  frame #5 {
                    n686 = local write "Ring 36"(u16 2 ("Ring 6")) -> ()
                    n687 = local write "Ring 35"(u16 0 ("Ring 5")) -> ()
                  }
                }
              }
              frame True {
                n688 = flat-sequence {
                  frame #0 {
                    n689 = local write "Ring 31"(u16 1 ("Ring 1")) -> ()
                    n690 = Wait (ms)(milliseconds to wait=u32 100) -> ()  [unwired: 1 out]
                  }
                  frame #1 {
                    n691 = local write "Ring 32"(u16 1 ("Ring 2")) -> ()
                    n692 = local write "Ring 31"(u16 0 ("Ring 1")) -> ()
                    n693 = Wait (ms)(milliseconds to wait=u32 100) -> ()  [unwired: 1 out]
                  }
                  frame #2 {
                    n694 = local write "Ring 33"(u16 1 ("Ring 3")) -> ()
                    n695 = local write "Ring 32"(u16 0 ("Ring 2")) -> ()
                    n696 = Wait (ms)(milliseconds to wait=u32 100) -> ()  [unwired: 1 out]
                  }
                  frame #3 {
                    n697 = local write "Ring 34"(u16 1 ("Ring 4")) -> ()
                    n698 = local write "Ring 33"(u16 0 ("Ring 3")) -> ()
                    n699 = Wait (ms)(milliseconds to wait=u32 100) -> ()  [unwired: 1 out]
                  }
                  frame #4 {
                    n700 = local write "Ring 35"(u16 1 ("Ring 5")) -> ()
                    n701 = local write "Ring 34"(u16 0 ("Ring 4")) -> ()
                    n702 = Wait (ms)(milliseconds to wait=u32 100) -> ()  [unwired: 1 out]
                  }
                  frame #5 {
                    n703 = local write "Ring 36"(u16 1 ("Ring 6")) -> ()
                    n704 = local write "Ring 35"(u16 0 ("Ring 5")) -> ()
                  }
                }
              }
            }
          }
          frame 2 {
            n705 = case shown="True" w708 {
              frame False {
                n706 = flat-sequence {
                  frame #0 {
                    n707 = local write "Ring 31"(u16 2 ("Ring 1")) -> ()
                    n708 = Wait (ms)(milliseconds to wait=u32 100) -> ()  [unwired: 1 out]
                  }
                  frame #1 {
                    n709 = local write "Ring 32"(u16 2 ("Ring 2")) -> ()
                    n710 = local write "Ring 31"(u16 0 ("Ring 1")) -> ()
                    n711 = Wait (ms)(milliseconds to wait=u32 100) -> ()  [unwired: 1 out]
                  }
                  frame #2 {
                    n712 = local write "Ring 33"(u16 2 ("Ring 3")) -> ()
                    n713 = local write "Ring 32"(u16 0 ("Ring 2")) -> ()
                    n714 = Wait (ms)(milliseconds to wait=u32 100) -> ()  [unwired: 1 out]
                  }
                  frame #3 {
                    n715 = local write "Ring 34"(u16 2 ("Ring 4")) -> ()
                    n716 = local write "Ring 33"(u16 0 ("Ring 3")) -> ()
                    n717 = Wait (ms)(milliseconds to wait=u32 100) -> ()  [unwired: 1 out]
                  }
                  frame #4 {
                    n718 = local write "Ring 35"(u16 2 ("Ring 5")) -> ()
                    n719 = local write "Ring 34"(u16 0 ("Ring 4")) -> ()
                  }
                }
              }
              frame True {
                n720 = flat-sequence {
                  frame #0 {
                    n721 = local write "Ring 31"(u16 1 ("Ring 1")) -> ()
                    n722 = Wait (ms)(milliseconds to wait=u32 100) -> ()  [unwired: 1 out]
                  }
                  frame #1 {
                    n723 = local write "Ring 32"(u16 1 ("Ring 2")) -> ()
                    n724 = local write "Ring 31"(u16 0 ("Ring 1")) -> ()
                    n725 = Wait (ms)(milliseconds to wait=u32 100) -> ()  [unwired: 1 out]
                  }
                  frame #2 {
                    n726 = local write "Ring 33"(u16 1 ("Ring 3")) -> ()
                    n727 = local write "Ring 32"(u16 0 ("Ring 2")) -> ()
                    n728 = Wait (ms)(milliseconds to wait=u32 100) -> ()  [unwired: 1 out]
                  }
                  frame #3 {
                    n729 = local write "Ring 34"(u16 1 ("Ring 4")) -> ()
                    n730 = local write "Ring 33"(u16 0 ("Ring 3")) -> ()
                    n731 = Wait (ms)(milliseconds to wait=u32 100) -> ()  [unwired: 1 out]
                  }
                  frame #4 {
                    n732 = local write "Ring 35"(u16 1 ("Ring 5")) -> ()
                    n733 = local write "Ring 34"(u16 0 ("Ring 4")) -> ()
                  }
                }
              }
            }
          }
          frame 3 {
            n734 = case shown="True" w736 {
              frame False {
                n735 = flat-sequence {
                  frame #0 {
                    n736 = local write "Ring 31"(u16 2 ("Ring 1")) -> ()
                    n737 = Wait (ms)(milliseconds to wait=u32 100) -> ()  [unwired: 1 out]
                  }
                  frame #1 {
                    n738 = local write "Ring 32"(u16 2 ("Ring 2")) -> ()
                    n739 = local write "Ring 31"(u16 0 ("Ring 1")) -> ()
                    n740 = Wait (ms)(milliseconds to wait=u32 100) -> ()  [unwired: 1 out]
                  }
                  frame #2 {
                    n741 = local write "Ring 33"(u16 2 ("Ring 3")) -> ()
                    n742 = local write "Ring 32"(u16 0 ("Ring 2")) -> ()
                    n743 = Wait (ms)(milliseconds to wait=u32 100) -> ()  [unwired: 1 out]
                  }
                  frame #3 {
                    n744 = local write "Ring 34"(u16 2 ("Ring 4")) -> ()
                    n745 = local write "Ring 33"(u16 0 ("Ring 3")) -> ()
                  }
                }
              }
              frame True {
                n746 = flat-sequence {
                  frame #0 {
                    n747 = local write "Ring 31"(u16 1 ("Ring 1")) -> ()
                    n748 = Wait (ms)(milliseconds to wait=u32 100) -> ()  [unwired: 1 out]
                  }
                  frame #1 {
                    n749 = local write "Ring 32"(u16 1 ("Ring 2")) -> ()
                    n750 = local write "Ring 31"(u16 0 ("Ring 1")) -> ()
                    n751 = Wait (ms)(milliseconds to wait=u32 100) -> ()  [unwired: 1 out]
                  }
                  frame #2 {
                    n752 = local write "Ring 33"(u16 1 ("Ring 3")) -> ()
                    n753 = local write "Ring 32"(u16 0 ("Ring 2")) -> ()
                    n754 = Wait (ms)(milliseconds to wait=u32 100) -> ()  [unwired: 1 out]
                  }
                  frame #3 {
                    n755 = local write "Ring 34"(u16 1 ("Ring 4")) -> ()
                    n756 = local write "Ring 33"(u16 0 ("Ring 3")) -> ()
                  }
                }
              }
            }
          }
          frame 4 {
            n757 = case shown="False" w758 {
              frame False {
                n758 = flat-sequence {
                  frame #0 {
                    n759 = local write "Ring 31"(u16 2 ("Ring 1")) -> ()
                    n760 = Wait (ms)(milliseconds to wait=u32 100) -> ()  [unwired: 1 out]
                  }
                  frame #1 {
                    n761 = local write "Ring 32"(u16 2 ("Ring 2")) -> ()
                    n762 = local write "Ring 31"(u16 0 ("Ring 1")) -> ()
                    n763 = Wait (ms)(milliseconds to wait=u32 100) -> ()  [unwired: 1 out]
                  }
                  frame #2 {
                    n764 = local write "Ring 33"(u16 2 ("Ring 3")) -> ()
                    n765 = local write "Ring 32"(u16 0 ("Ring 2")) -> ()
                  }
                }
              }
              frame True {
                n766 = flat-sequence {
                  frame #0 {
                    n767 = local write "Ring 31"(u16 1 ("Ring 1")) -> ()
                    n768 = Wait (ms)(milliseconds to wait=u32 100) -> ()  [unwired: 1 out]
                  }
                  frame #1 {
                    n769 = local write "Ring 32"(u16 1 ("Ring 2")) -> ()
                    n770 = local write "Ring 31"(u16 0 ("Ring 1")) -> ()
                    n771 = Wait (ms)(milliseconds to wait=u32 100) -> ()  [unwired: 1 out]
                  }
                  frame #2 {
                    n772 = local write "Ring 33"(u16 1 ("Ring 3")) -> ()
                    n773 = local write "Ring 32"(u16 0 ("Ring 2")) -> ()
                  }
                }
              }
            }
          }
          frame 5 {
            n774 = case shown="False" w774 {
              frame False {
                n775 = flat-sequence {
                  frame #0 {
                    n776 = local write "Ring 31"(u16 2 ("Ring 1")) -> ()
                    n777 = Wait (ms)(milliseconds to wait=u32 100) -> ()  [unwired: 1 out]
                  }
                  frame #1 {
                    n778 = local write "Ring 32"(u16 2 ("Ring 2")) -> ()
                    n779 = local write "Ring 31"(u16 0 ("Ring 1")) -> ()
                  }
                }
              }
              frame True {
                n780 = flat-sequence {
                  frame #0 {
                    n781 = local write "Ring 31"(u16 1 ("Ring 1")) -> ()
                    n782 = Wait (ms)(milliseconds to wait=u32 100) -> ()  [unwired: 1 out]
                  }
                  frame #1 {
                    n783 = local write "Ring 32"(u16 1 ("Ring 2")) -> ()
                    n784 = local write "Ring 31"(u16 0 ("Ring 1")) -> ()
                  }
                }
              }
            }
          }
          frame 6 {
            n785 = case shown="False" w784 {
              frame False {
                n786 = flat-sequence {
                  frame #0 {
                    n787 = local write "Ring 31"(u16 2 ("Ring 1")) -> ()
                  }
                }
              }
              frame True {
                n788 = flat-sequence {
                  frame #0 {
                    n789 = local write "Ring 31"(u16 1 ("Ring 1")) -> ()
                  }
                }
              }
            }
          }
        }
        n790 = Not(x=w668) -> (.not. x?=w667:bool)
      }
      event "col7": Mouse Down {
        n791 = event-data() -> ()  [unwired: 1 in, 8 out]
        n792 = Add(x=w798, y=1) -> (x+y=w797:i32)
        n793 = case shown="6" w797 {
          selector: w797 -> [w800 w802 w836 w864 w886 w902 w912]
          tunnel: [w800 w802 w836 w864 w886 w902 w912] -> w796
          tunnel: w788 -> [_ w801 w835 w863 w885 w901 w911]
          frame 0, Default {
          }
          frame 1 {
            n794 = case shown="True" w801 {
              frame False {
                n795 = flat-sequence {
                  frame #0 {
                    n796 = local write "Ring 37"(u16 2 ("Ring 1")) -> ()
                    n797 = Wait (ms)(milliseconds to wait=u32 100) -> ()  [unwired: 1 out]
                  }
                  frame #1 {
                    n798 = local write "Ring 38"(u16 2 ("Ring 2")) -> ()
                    n799 = local write "Ring 37"(u16 0 ("Ring 1")) -> ()
                    n800 = Wait (ms)(milliseconds to wait=u32 100) -> ()  [unwired: 1 out]
                  }
                  frame #2 {
                    n801 = local write "Ring 39"(u16 2 ("Ring 3")) -> ()
                    n802 = local write "Ring 38"(u16 0 ("Ring 2")) -> ()
                    n803 = Wait (ms)(milliseconds to wait=u32 100) -> ()  [unwired: 1 out]
                  }
                  frame #3 {
                    n804 = local write "Ring 40"(u16 2 ("Ring 4")) -> ()
                    n805 = local write "Ring 39"(u16 0 ("Ring 3")) -> ()
                    n806 = Wait (ms)(milliseconds to wait=u32 100) -> ()  [unwired: 1 out]
                  }
                  frame #4 {
                    n807 = local write "Ring 41"(u16 2 ("Ring 5")) -> ()
                    n808 = local write "Ring 40"(u16 0 ("Ring 4")) -> ()
                    n809 = Wait (ms)(milliseconds to wait=u32 100) -> ()  [unwired: 1 out]
                  }
                  frame #5 {
                    n810 = local write "Ring 42"(u16 2 ("Ring 6")) -> ()
                    n811 = local write "Ring 41"(u16 0 ("Ring 5")) -> ()
                  }
                }
              }
              frame True {
                n812 = flat-sequence {
                  frame #0 {
                    n813 = local write "Ring 37"(u16 1 ("Ring 1")) -> ()
                    n814 = Wait (ms)(milliseconds to wait=u32 100) -> ()  [unwired: 1 out]
                  }
                  frame #1 {
                    n815 = local write "Ring 38"(u16 1 ("Ring 2")) -> ()
                    n816 = local write "Ring 37"(u16 0 ("Ring 1")) -> ()
                    n817 = Wait (ms)(milliseconds to wait=u32 100) -> ()  [unwired: 1 out]
                  }
                  frame #2 {
                    n818 = local write "Ring 39"(u16 1 ("Ring 3")) -> ()
                    n819 = local write "Ring 38"(u16 0 ("Ring 2")) -> ()
                    n820 = Wait (ms)(milliseconds to wait=u32 100) -> ()  [unwired: 1 out]
                  }
                  frame #3 {
                    n821 = local write "Ring 40"(u16 1 ("Ring 4")) -> ()
                    n822 = local write "Ring 39"(u16 0 ("Ring 3")) -> ()
                    n823 = Wait (ms)(milliseconds to wait=u32 100) -> ()  [unwired: 1 out]
                  }
                  frame #4 {
                    n824 = local write "Ring 41"(u16 1 ("Ring 5")) -> ()
                    n825 = local write "Ring 40"(u16 0 ("Ring 4")) -> ()
                    n826 = Wait (ms)(milliseconds to wait=u32 100) -> ()  [unwired: 1 out]
                  }
                  frame #5 {
                    n827 = local write "Ring 42"(u16 1 ("Ring 6")) -> ()
                    n828 = local write "Ring 41"(u16 0 ("Ring 5")) -> ()
                  }
                }
              }
            }
          }
          frame 2 {
            n829 = case shown="False" w835 {
              frame False {
                n830 = flat-sequence {
                  frame #0 {
                    n831 = local write "Ring 37"(u16 2 ("Ring 1")) -> ()
                    n832 = Wait (ms)(milliseconds to wait=u32 100) -> ()  [unwired: 1 out]
                  }
                  frame #1 {
                    n833 = local write "Ring 38"(u16 2 ("Ring 2")) -> ()
                    n834 = local write "Ring 37"(u16 0 ("Ring 1")) -> ()
                    n835 = Wait (ms)(milliseconds to wait=u32 100) -> ()  [unwired: 1 out]
                  }
                  frame #2 {
                    n836 = local write "Ring 39"(u16 2 ("Ring 3")) -> ()
                    n837 = local write "Ring 38"(u16 0 ("Ring 2")) -> ()
                    n838 = Wait (ms)(milliseconds to wait=u32 100) -> ()  [unwired: 1 out]
                  }
                  frame #3 {
                    n839 = local write "Ring 40"(u16 2 ("Ring 4")) -> ()
                    n840 = local write "Ring 39"(u16 0 ("Ring 3")) -> ()
                    n841 = Wait (ms)(milliseconds to wait=u32 100) -> ()  [unwired: 1 out]
                  }
                  frame #4 {
                    n842 = local write "Ring 41"(u16 2 ("Ring 5")) -> ()
                    n843 = local write "Ring 40"(u16 0 ("Ring 4")) -> ()
                  }
                }
              }
              frame True {
                n844 = flat-sequence {
                  frame #0 {
                    n845 = local write "Ring 37"(u16 1 ("Ring 1")) -> ()
                    n846 = Wait (ms)(milliseconds to wait=u32 100) -> ()  [unwired: 1 out]
                  }
                  frame #1 {
                    n847 = local write "Ring 38"(u16 1 ("Ring 2")) -> ()
                    n848 = local write "Ring 37"(u16 0 ("Ring 1")) -> ()
                    n849 = Wait (ms)(milliseconds to wait=u32 100) -> ()  [unwired: 1 out]
                  }
                  frame #2 {
                    n850 = local write "Ring 39"(u16 1 ("Ring 3")) -> ()
                    n851 = local write "Ring 38"(u16 0 ("Ring 2")) -> ()
                    n852 = Wait (ms)(milliseconds to wait=u32 100) -> ()  [unwired: 1 out]
                  }
                  frame #3 {
                    n853 = local write "Ring 40"(u16 1 ("Ring 4")) -> ()
                    n854 = local write "Ring 39"(u16 0 ("Ring 3")) -> ()
                    n855 = Wait (ms)(milliseconds to wait=u32 100) -> ()  [unwired: 1 out]
                  }
                  frame #4 {
                    n856 = local write "Ring 41"(u16 1 ("Ring 5")) -> ()
                    n857 = local write "Ring 40"(u16 0 ("Ring 4")) -> ()
                  }
                }
              }
            }
          }
          frame 3 {
            n858 = case shown="False" w863 {
              frame False {
                n859 = flat-sequence {
                  frame #0 {
                    n860 = local write "Ring 37"(u16 2 ("Ring 1")) -> ()
                    n861 = Wait (ms)(milliseconds to wait=u32 100) -> ()  [unwired: 1 out]
                  }
                  frame #1 {
                    n862 = local write "Ring 38"(u16 2 ("Ring 2")) -> ()
                    n863 = local write "Ring 37"(u16 0 ("Ring 1")) -> ()
                    n864 = Wait (ms)(milliseconds to wait=u32 100) -> ()  [unwired: 1 out]
                  }
                  frame #2 {
                    n865 = local write "Ring 39"(u16 2 ("Ring 3")) -> ()
                    n866 = local write "Ring 38"(u16 0 ("Ring 2")) -> ()
                    n867 = Wait (ms)(milliseconds to wait=u32 100) -> ()  [unwired: 1 out]
                  }
                  frame #3 {
                    n868 = local write "Ring 40"(u16 2 ("Ring 4")) -> ()
                    n869 = local write "Ring 39"(u16 0 ("Ring 3")) -> ()
                  }
                }
              }
              frame True {
                n870 = flat-sequence {
                  frame #0 {
                    n871 = local write "Ring 37"(u16 1 ("Ring 1")) -> ()
                    n872 = Wait (ms)(milliseconds to wait=u32 100) -> ()  [unwired: 1 out]
                  }
                  frame #1 {
                    n873 = local write "Ring 38"(u16 1 ("Ring 2")) -> ()
                    n874 = local write "Ring 37"(u16 0 ("Ring 1")) -> ()
                    n875 = Wait (ms)(milliseconds to wait=u32 100) -> ()  [unwired: 1 out]
                  }
                  frame #2 {
                    n876 = local write "Ring 39"(u16 1 ("Ring 3")) -> ()
                    n877 = local write "Ring 38"(u16 0 ("Ring 2")) -> ()
                    n878 = Wait (ms)(milliseconds to wait=u32 100) -> ()  [unwired: 1 out]
                  }
                  frame #3 {
                    n879 = local write "Ring 40"(u16 1 ("Ring 4")) -> ()
                    n880 = local write "Ring 39"(u16 0 ("Ring 3")) -> ()
                  }
                }
              }
            }
          }
          frame 4 {
            n881 = case shown="True" w885 {
              frame False {
                n882 = flat-sequence {
                  frame #0 {
                    n883 = local write "Ring 37"(u16 2 ("Ring 1")) -> ()
                    n884 = Wait (ms)(milliseconds to wait=u32 100) -> ()  [unwired: 1 out]
                  }
                  frame #1 {
                    n885 = local write "Ring 38"(u16 2 ("Ring 2")) -> ()
                    n886 = local write "Ring 37"(u16 0 ("Ring 1")) -> ()
                    n887 = Wait (ms)(milliseconds to wait=u32 100) -> ()  [unwired: 1 out]
                  }
                  frame #2 {
                    n888 = local write "Ring 39"(u16 2 ("Ring 3")) -> ()
                    n889 = local write "Ring 38"(u16 0 ("Ring 2")) -> ()
                  }
                }
              }
              frame True {
                n890 = flat-sequence {
                  frame #0 {
                    n891 = local write "Ring 37"(u16 1 ("Ring 1")) -> ()
                    n892 = Wait (ms)(milliseconds to wait=u32 100) -> ()  [unwired: 1 out]
                  }
                  frame #1 {
                    n893 = local write "Ring 38"(u16 1 ("Ring 2")) -> ()
                    n894 = local write "Ring 37"(u16 0 ("Ring 1")) -> ()
                    n895 = Wait (ms)(milliseconds to wait=u32 100) -> ()  [unwired: 1 out]
                  }
                  frame #2 {
                    n896 = local write "Ring 39"(u16 1 ("Ring 3")) -> ()
                    n897 = local write "Ring 38"(u16 0 ("Ring 2")) -> ()
                  }
                }
              }
            }
          }
          frame 5 {
            n898 = case shown="True" w901 {
              frame False {
                n899 = flat-sequence {
                  frame #0 {
                    n900 = local write "Ring 37"(u16 2 ("Ring 1")) -> ()
                    n901 = Wait (ms)(milliseconds to wait=u32 100) -> ()  [unwired: 1 out]
                  }
                  frame #1 {
                    n902 = local write "Ring 38"(u16 2 ("Ring 2")) -> ()
                    n903 = local write "Ring 37"(u16 0 ("Ring 1")) -> ()
                  }
                }
              }
              frame True {
                n904 = flat-sequence {
                  frame #0 {
                    n905 = local write "Ring 37"(u16 1 ("Ring 1")) -> ()
                    n906 = Wait (ms)(milliseconds to wait=u32 100) -> ()  [unwired: 1 out]
                  }
                  frame #1 {
                    n907 = local write "Ring 38"(u16 1 ("Ring 2")) -> ()
                    n908 = local write "Ring 37"(u16 0 ("Ring 1")) -> ()
                  }
                }
              }
            }
          }
          frame 6 {
            n909 = case shown="True" w911 {
              frame False {
                n910 = flat-sequence {
                  frame #0 {
                    n911 = local write "Ring 37"(u16 2 ("Ring 1")) -> ()
                  }
                }
              }
              frame True {
                n912 = flat-sequence {
                  frame #0 {
                    n913 = local write "Ring 37"(u16 1 ("Ring 1")) -> ()
                  }
                }
              }
            }
          }
        }
        n914 = Not(x=w788) -> (.not. x?=w789:bool)
      }
      event "Ring 1", "Ring 2", "Ring 3", "Ring 4", "Ring 5", "Ring 6", "Ring 7", "Ring 8", "Ring 9", "Ring 10", "Ring 11", "Ring 12", "Ring 13", "Ring 14", "Ring 15", "Ring 16", "Ring 17", "Ring 18", "Ring 19", "Ring 20", "Ring 21", "Ring 22", "Ring 23", "Ring 24", "Ring 25", "Ring 26", "Ring 27", "Ring 28", "Ring 29", "Ring 30", "Ring 31", "Ring 32", "Ring 33", "Ring 34", "Ring 35", "Ring 36", "Ring 37", "Ring 38", "Ring 39", "Ring 40", "Ring 41", "Ring 42": Mouse Down? {
        n915 = event-data() -> ()  [unwired: 1 in, 8 out]
        n916 = event-data("Discard?"=TRUE) -> ()  [unwired: 4 in, 1 out]
      }
      event "OK Button": Value Change {
        w930 = u16 0 ("Ring 42")
        w929 = u16 0 ("Ring 36")
        w928 = u16 0 ("Ring 30")
        w927 = u16 0 ("Ring 24")
        w926 = u16 0 ("Ring 18")
        w925 = u16 0 ("Ring 12")
        w924 = 0
        n917 = event-data() -> ()  [unwired: 1 in, 6 out]
        n918 = local write "Ring 6"(w924) -> ()
        n919 = local write "Ring 5"(w924) -> ()
        n920 = local write "Ring 4"(w924) -> ()
        n921 = local write "Ring 3"(w924) -> ()
        n922 = local write "Ring 2"(w924) -> ()
        n923 = local write "Ring 1"(w924) -> ()
        n924 = local write "Ring 42"(w930) -> ()
        n925 = local write "Ring 41"(w930) -> ()
        n926 = local write "Ring 40"(w930) -> ()
        n927 = local write "Ring 39"(w930) -> ()
        n928 = local write "Ring 38"(w930) -> ()
        n929 = local write "Ring 37"(w930) -> ()
        n930 = local write "Ring 36"(w929) -> ()
        n931 = local write "Ring 35"(w929) -> ()
        n932 = local write "Ring 34"(w929) -> ()
        n933 = local write "Ring 33"(w929) -> ()
        n934 = local write "Ring 32"(w929) -> ()
        n935 = local write "Ring 31"(w929) -> ()
        n936 = local write "Ring 30"(w928) -> ()
        n937 = local write "Ring 29"(w928) -> ()
        n938 = local write "Ring 28"(w928) -> ()
        n939 = local write "Ring 27"(w928) -> ()
        n940 = local write "Ring 26"(w928) -> ()
        n941 = local write "Ring 25"(w928) -> ()
        n942 = local write "Ring 24"(w927) -> ()
        n943 = local write "Ring 23"(w927) -> ()
        n944 = local write "Ring 22"(w927) -> ()
        n945 = local write "Ring 21"(w927) -> ()
        n946 = local write "Ring 20"(w927) -> ()
        n947 = local write "Ring 19"(w927) -> ()
        n948 = local write "Ring 18"(w926) -> ()
        n949 = local write "Ring 17"(w926) -> ()
        n950 = local write "Ring 16"(w926) -> ()
        n951 = local write "Ring 15"(w926) -> ()
        n952 = local write "Ring 14"(w926) -> ()
        n953 = local write "Ring 13"(w926) -> ()
        n954 = local write "Ring 9"(w925) -> ()
        n955 = local write "Ring 8"(w925) -> ()
        n956 = local write "Ring 7"(w925) -> ()
        n957 = local write "Ring 11"(w925) -> ()
        n958 = local write "Ring 10"(w925) -> ()
        n959 = local write "Ring 12"(w925) -> ()
      }
    }
  }
